vi "imp_test_v10_2.vi"() -> ()   [LabVIEW 2014]
uses:
  <vilib>/LabVIEW Targets/FPGA/cRIO/shared/nicrio_ModuleControls/nicrio_cRIO-9237_DataRatesRing.ctl
  <vilib>/LabVIEW Targets/FPGA/cRIO/shared/nicrio_ModuleControls/nicrio_cRIO-9237_ExcitationVoltageRing.ctl
  <vilib>/rvi/FXPMathLib/FxpSinAndCos/subVIs/nifxpmath_SinAndCos_SimConfig.ctl
  <vilib>/rvi/Emulation/niFpgaGetClockAttributes.vi
  <vilib>/rvi/Emulation/niFpgaSctlEmulationGetInTimedLoop.vi
  <vilib>/rvi/Emulation/niFpgaEmulationReportErrorSimple.vi
  <vilib>/rvi/Emulation/niFpgaProcessEmulError.vi
  <vilib>/rvi/interface/RandomDataEmulation/nirviRandomDataMultiElementFPGAFIFO.vi
  <instcachedir>/0/nirviRandomDataMultiElementFPGAFIFO_AD0CFC12EF974623A9C2E4184BC062B2.lvgen/nirviRandomDataMultiElementFPGAFIFO_AD0CFC12EF974623A9C2E4184BC062B2_010.vi
  <vilib>/rvi/interface/RandomDataEmulation/niFpgaRandomDataHandleErrors.vi
  <vilib>/rvi/Emulation/niFpgaCriticalErrorInLSC.vi
  <vilib>/rvi/FXPMathLib/FxpSinAndCos/simVIs/DllFxpSinAndCosTemp_sub.vi
  <vilib>/rvi/eio/common/nirviEmuTemplateMethod_errors.vi
  <vilib>/rvi/eio/common/nirviEmuTemplatePropertySet_errors.vi
  <vilib>/rvi/DataTransferAndStorage/Container/XNode/niFpgaContainer.xnode
  <vilib>/rvi/interface/RandomDataEmulation/nirviRandomDataFpgaMultiElementTemplate.vi
  <vilib>/rvi/FXPMathLib/FxpSinAndCos/XNode/nifxpmath_SinAndCos.xnode
  <vilib>/eio/EIONode/EIONode.xnode
  <vilib>/rvi/Analysis/measure/butterworth/XNode/niFpgaButterworthFilter.xnode
  <vilib>/eio/EIOPropertyNode/EIOPropertyNode.xnode
  <vilib>/rvi/eio/common/nirviEmuTemplatePropertyGet_errors.vi
  <vilib>/rvi/eio/common/nirviEmuTemplatePropertyGet_noerrors.vi
  <vilib>/rvi/eio/common/nirviEmuTemplatePropertySet_noerrors.vi
panel:
  in  "F_Threshold_p":fxp<+,12,4>
  in  "F_Threshold_y":fxp<+,12,4>
  out "omega_y (Mavg)":fxp<+/-,36,13>
  out "Dy_d (Mavg)":fxp<+/-,36,13>
  out "omega_p (Mavg)":fxp<+/-,36,13>
  out "Dp_d (Mavg)":fxp<+/-,36,13>
  out "omega_p2 (Mavg)":fxp<+/-,36,14>
  out "Dp2_d (Mavg)":fxp<+/-,36,14>
  out "omega_y2 (Mavg)":fxp<+/-,36,14>
  out "Dy2_d (Mavg)":fxp<+/-,36,14>
  in  "mt0_y2":u32
  in  "mt0_p2":u32
  out "Dy_d (Mavg w. f.)":fxp<+/-,36,14>
  out "Dp_d (Mavg w. f.)":fxp<+/-,36,14>
  in  "Dp_d (Mavg) coeff.":i32[](array[numeric])=[946630756, 63555534]
  in  "Dy_d (Mavg) coeff.":i32[](array[numeric])=[946630756, 63555534]
  out "omega_y (Mavg w. f.)":fxp<+/-,36,14>
  in  "omega_y(Mavg) coeff.":i32[](array[numeric])=[946630756, 63555534]
  out "omega_p (Mavg w. f)":fxp<+/-,36,14>
  in  "omega_P(Mavg) coeff.":i32[](array[numeric])=[946630756, 63555534]
  out "PID (kHz)":fxp<+/-,20,10>
  in  "Set 6":bool
  in  "Set 5":bool
  in  "Set 4":bool
  in  "Set 3":bool
  in  "Set 2":bool
  in  "Set 1":bool
  out "Dy1_d (T)":fxp<+/-,36,13>
  out "omega_y1 (T)":fxp<+/-,36,13>
  out "Dp1_d (T)":fxp<+/-,36,13>
  out "omega_p1 (T)":fxp<+/-,36,13>
  out "Dy2_d (T)":fxp<+/-,36,13>
  out "Dp2_d (T)":fxp<+/-,36,13>
  out "omega_y2 (T)":fxp<+/-,36,13>
  out "omega_p2 (T)":fxp<+/-,36,13>
  out "mt_omega_y2":u32
  out "mt_omega_p2":u32
  out "rad_y2":fxp<+/-,33,20>
  out "D_y2":fxp<+/-,32,7>
  out "rad_y1":fxp<+/-,33,20>
  out "D_y1":fxp<+/-,32,7>
  out "Encoder Position_y1":i32
  out "Encoder Position_y2":i32
  out "Encoder Position_p2":i32
  out "D_p2":fxp<+/-,32,7>
  out "rad_p2":fxp<+/-,33,20>
  out "D_p1":fxp<+/-,32,7>
  out "rad_p1":fxp<+/-,33,20>
  out "Encoder Position_p1":i32
  in  "Mag. factor_y":fxp<+/-,20,3>
  in  "Mag. encoder_y":bool
  out "omega_y (rad/s)":fxp<+/-,36,13>
  out "Dy_d (mm/s)":fxp<+/-,36,13>
  in  "Vy. Est.":i16(ring) items=["T", "Mavg", "Mavg w. f."]
  out "omega_y1 (Mavg)":fxp<+/-,36,14>
  out "Dy1_d (Mavg)":fxp<+/-,36,14>
  in  "Dy_d_M_avg_Tc (uSec)":i32
  out "Dp1_d (Mavg)":fxp<+/-,36,14>
  out "omega_p1 (Mavg)":fxp<+/-,36,14>
  in  "Dp_d_M_avg_Tc (uSec)":i32
  out "Dp_d (T)":fxp<+/-,36,13>
  out "omega_p (T)":fxp<+/-,36,13>
  in  "Vp. Est.":i16(ring) items=["T", "Mavg", "Mavg w. f."]
  in  "Mag. factor_p":fxp<+/-,20,3>
  in  "Mag. encoder_p":bool
  in  "Belt_out_p":fxp<+/-,7,7>
  in  "Belt_in_p":fxp<+/-,6,6>
  in  "Belt_out_y":fxp<+/-,7,7>
  in  "Belt_in_y":fxp<+/-,6,6>
  out "Fp_dc":fxp<+/-,32,10>
  out "Fy_dc":fxp<+/-,32,10>
  in  "Zero_y":bool
  in  "Zero_p":bool
  in  "mt0_p1":u32
  in  "Encoder reset":bool
  out "fpt_d":fxp<+/-,36,18>
  out "Dp_error_dd":fxp<+/-,36,16>
  out "Dp_error_d":fxp<+/-,33,8>
  in  "Dp_dd coeff.":i32[](array[numeric])=[946630756, 63555534]
  out "Dp_dd":fxp<+/-,36,25>
  out "dFp_PID":fxp<+/-,36,18>
  in  "dFp_PID coeff.":i32[](array[numeric])=[946630756, 63555534]
  out "fpt_i":fxp<+/-,34,18>
  in  "Bv_p":fxp<+/-,22,8>
  in  "Kv_p":fxp<+/-,22,8>
  out "Dp_error":fxp<+/-,22,7>
  out "Dpr_sin":fxp<+/-,22,7>
  in  "Sin offset_p":fxp<+/-,22,7>
  in  "Sin magnitude_p":fxp<+/-,21,6>
  out "Dpr_sin_dd":fxp<+/-,35,20>
  out "Dpr_sin_d":fxp<+/-,33,15>
  out "Sin omega_p":fxp<+/-,34,9>
  in  "Sin wave freq._p (Hz)":fxp<+/-,32,6>
  in  "Dpr_step":fxp<+/-,22,7>
  out "Dpr_for":fxp<+/-,22,7>
  in  "Command_p":i16(ring) items=["Step", "Sine"]
  in  "Ki_p":fxp<+/-,30,9>
  out "Fp_PID":fxp<+/-,36,16>
  in  "fp_tolorance":fxp<+,22,6>
  out "fp_tilde":fxp<+/-,33,10>
  in  "Kd_p":fxp<+/-,30,9>
  in  "Kp_p":fxp<+/-,32,13>
  out "Fr_p":fxp<+/-,32,10>
  in  "S/F coeff_p":fxp<+/-,25,-10>
  in  "S/F coeff_y":fxp<+/-,25,-10>
  out "va_p":fxp<+/-,36,7>
  out "vb_p":fxp<+/-,37,8>
  out "vq_p_F":fxp<+/-,20,5> format="%.57g"
  out "vd_p_F":fxp<+/-,20,5>
  in  "dFp_add":bool
  in  "Stop motor_p":bool
  out "Force_p":fxp<+/-,32,10>
  in  "Strain selection_p":i16(ring) items=["Raw", "Avg.8", "Avg.8 w. filter"]
  out "Strain_p (Avg8 w. f)":fxp<+/-,36,8>
  in  "Strain_p Avg.8 coeff.":i32[](array[numeric])=[946630756, 63555534]
  out "Strain_p (Avg8)":fxp<+/-,36,4>
  out "Raw Strain_p":fxp<+/-,36,4>
  out "Mod6/AI3":fxp<+/-,36,4>
  in  "Strain gage reset_p":bool
  out "Dp_d (mm/s)":fxp<+/-,36,13>
  out "omega_p (rad/s)":fxp<+/-,36,13>
  out "mt_omega_p1":u32
  out "rad_p(NrTheta)":fxp<+/-,33,20>
  out "D_p(mm)":fxp<+/-,32,7>
  out "Encoder Position_p":i32
  in  "Encoder reset_p":bool
  out "Strain_y (Avg8 w. f)":fxp<+/-,36,8>
  in  "Strain_y Avg8 coeff.":i32[](array[numeric])=[-898916953, 1957103773, 3888751]
  out "Dyr_for":fxp<+/-,22,7>
  in  "Command_y":i16(ring) items=["Step", "Sine"]
  out "Strain_y (Avg8)":fxp<+/-,36,4>
  in  "Strain selection_y":i16(ring) items=["Raw", "Avg.8", "Avg.8 w. filter"]
  out "vb_y":fxp<+/-,38,8>
  out "va_y":fxp<+/-,38,8>
  out "fyt_d":fxp<+/-,36,18>
  out "Fr_y":fxp<+/-,32,10>
  in  "Bv_y":fxp<+/-,22,8>
  out "Dy_error_dd":fxp<+/-,36,16>
  out "Dy_error_d":fxp<+/-,33,8>
  in  "Kv_y":fxp<+/-,22,8>
  out "Dy_error":fxp<+/-,22,7>
  out "Dyr_sin_dd":fxp<+/-,35,20>
  out "Dyr_sin_d":fxp<+/-,33,15>
  out "Sin omega_y":fxp<+/-,34,9>
  out "Dyr_sin":fxp<+/-,22,7>
  in  "Sin offset_y":fxp<+/-,22,7>
  in  "Sin magnitude_y":fxp<+/-,21,6>
  out "Time now(s)":fxp<+,52,14>
  in  "Sin wave freq._y (Hz)":fxp<+/-,32,6>
  in  "Dyr_step":fxp<+/-,22,7>
  in  "Drive mode":i16(ring) items=["Backward", "Forward"]
  out "Dy_dd":fxp<+/-,36,25>
  in  "Dy_dd coeff.":i32[](array[numeric])=[946630756, 63555534]
  out "dFy_PID":fxp<+/-,36,18>
  in  "dFy_PID coeff.":i32[](array[numeric])=[946630756, 63555534]
  out "fyt_i":fxp<+/-,36,16>
  out "Fy_PID":fxp<+/-,36,16>
  in  "fy_tolorance":fxp<+,22,6>
  in  "Ki_y":fxp<+/-,30,9>
  in  "Kd_y":fxp<+/-,30,9>
  out "fy_tilde":fxp<+/-,32,10>
  in  "Kp_y":fxp<+/-,32,13>
  out "vq_y_F":fxp<+/-,20,5> format="%.57g"
  out "vd_y_F":fxp<+/-,20,5>
  in  "dFy_add":bool
  in  "Stop motor_y":bool
  out "Dy_d (T)":fxp<+/-,36,13>
  out "omega_y (T)":fxp<+/-,36,13>
  in  "mt0_y1":u32
  out "mt_omega_y1":u32
  out "rad_y(NrTheta)":fxp<+/-,33,20>
  out "D_y(mm)":fxp<+/-,32,7>
  out "Encoder Position_y":i32
  in  "Encoder reset_y":bool
  in  "Ini coe.":bool
  out "Loop rate (kHz)":fxp<+/-,36,7>
  out "Force_y":fxp<+/-,32,10>
  out "Raw Strain_y":fxp<+/-,36,4>
  in  "Strain gage reset_y":bool
  in  "Stop (Strain)":bool
  out "Mod6/AI2":fxp<+/-,36,4>
  in  "Excitation Voltage":T1 items=["2.5 Volts", "3.3 Volts", "5.0 Volts", "10.0 Volts", "External Excitation"]
  in  "Data Rate":T2=1 items=["50.000 kS/s (NI 9237)"=1, "25.000 kS/s (NI 9237)"=2, "16.667 kS/s (NI 9237)"=3, "12.500 kS/s (NI 9237)"=4, "10.000 kS/s (NI 9237)"=5, "8.333 kS/s (NI 9237)"=6, "7.143 kS/s (NI 9237)"=7, "6.250 kS/s (NI 9237)"=8, "5.556 kS/s (NI 9237)"=9, "5.000 kS/s (NI 9237)"=10, "4.545 kS/s (NI 9237)"=11, "4.167 kS/s (NI 9237)"=12, "3.846 kS/s (NI 9237)"=13, "3.571 kS/s (NI 9237)"=14, "3.333 kS/s (NI 9237)"=15, "3.125 kS/s (NI 9237)"=16, "2.941 kS/s (NI 9237)"=17, "2.778 kS/s (NI 9237)"=18, "2.632 kS/s (NI 9237)"=19, "2.500 kS/s (NI 9237)"=20, "2.381 kS/s (NI 9237)"=21, "2.273 kS/s (NI 9237)"=22, "2.174 kS/s (NI 9237)"=23, "2.083 kS/s (NI 9237)"=24, "2.000 kS/s (NI 9237)"=25, "1.923 kS/s (NI 9237)"=26, "1.852 kS/s (NI 9237)"=27, "1.786 kS/s (NI 9237)"=28, "1.724 kS/s (NI 9237)"=29, "1.667 kS/s (NI 9237)"=30, "1.613 kS/s (NI 9237)"=31]
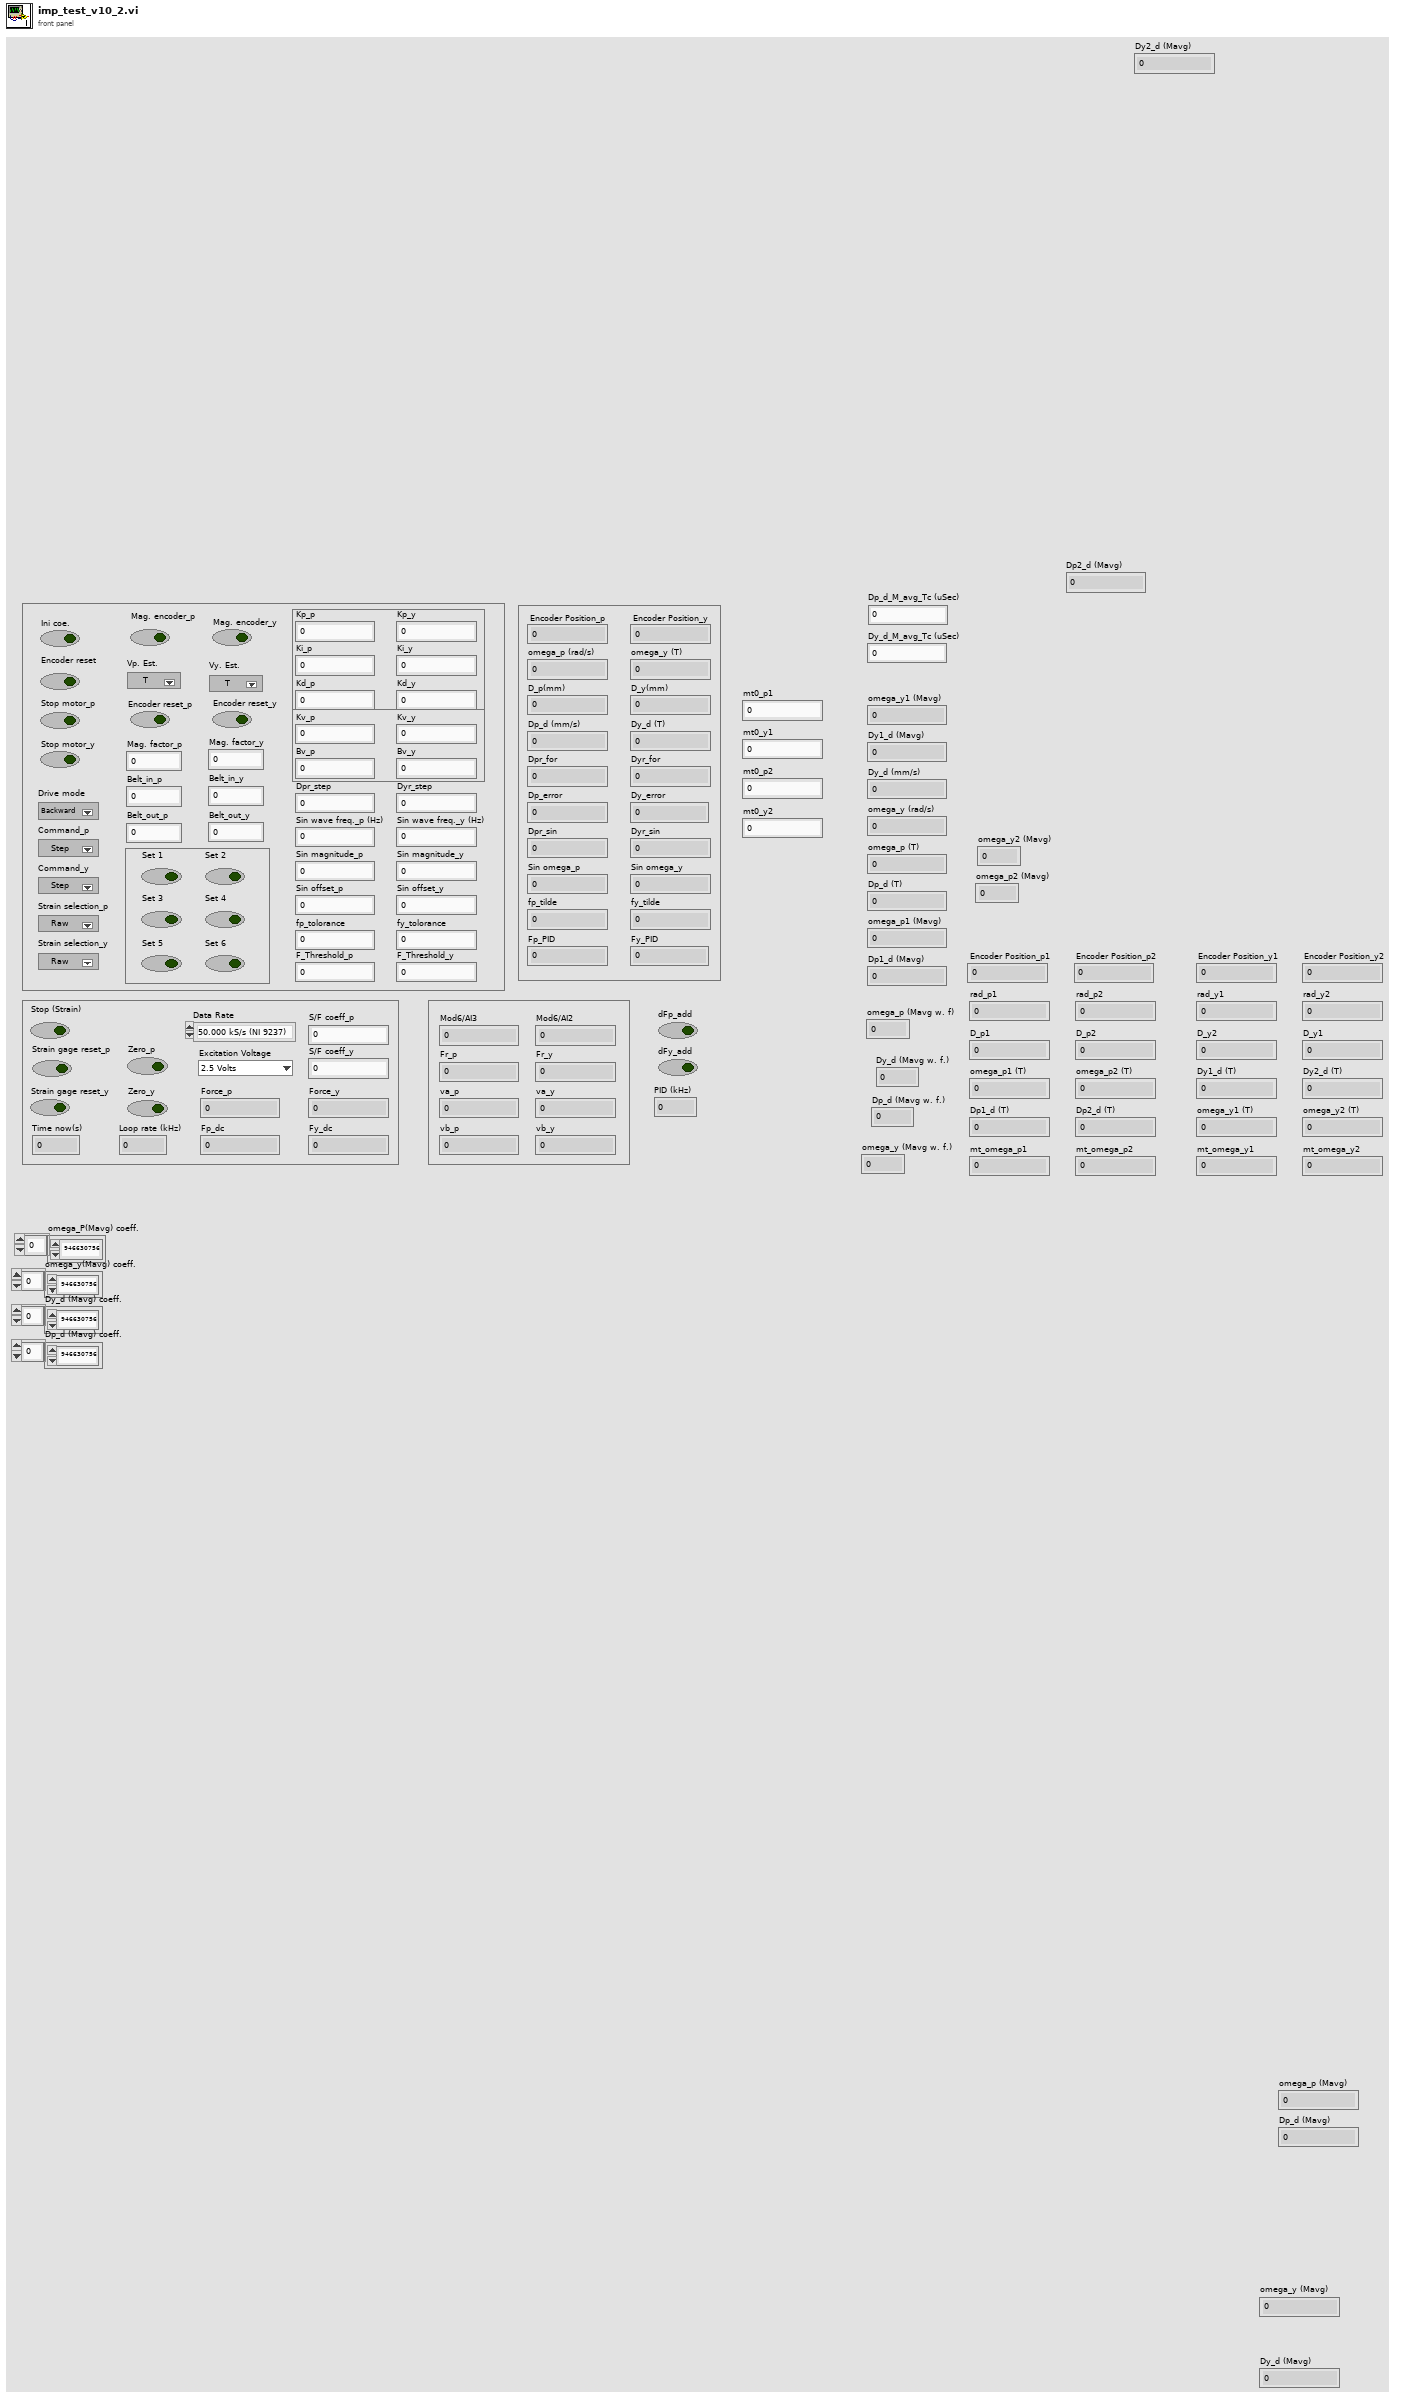
[diagram p1: front panel]
types:
  T1 = typedef "nicrio_cRIO-9237_ExcitationVoltageRing.ctl" = u8
  T2 = typedef "nicrio_cRIO-9237_DataRatesRing.ctl" = u8
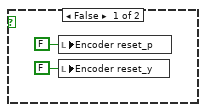
[diagram p12: hidden frame]
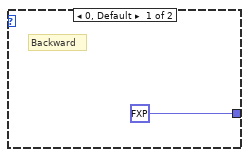
[diagram p13: hidden frame]
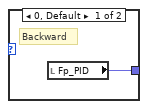
[diagram p14: hidden frame]
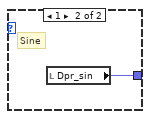
[diagram p15: hidden frame]
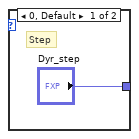
[diagram p16: hidden frame]
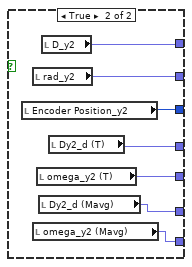
[diagram p17: hidden frame]
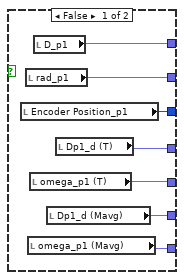
[diagram p18: hidden frame]
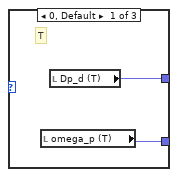
[diagram p19: hidden frame]
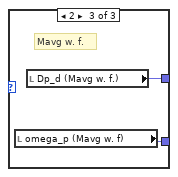
[diagram p20: hidden frame]
diagram:
  w2 = 25
  w5 = i16 25
  w13 = 25
  w16 = 25
  w21 = TRUE ("Half-Bridge Enable")
  # "rad_x2那邊:數據叫出來/8才會和馬達編碼器的rad一樣??"
  # "Encoder 4096ppr\nomega = 61359.2315154/mt\nomega0 = 2*pi/4096 (rad/s)"
  # "Encoder 800ppr\nomega = 314159.265359/mt\nomega0 = 2*pi/800 (rad/s)"
  # "v9\nKp改32/13\nKd改30/9\nKo改30/9"
  # "Resolutuin of Mag. Encoder = 4096*(F_mag)"
  # "use Mavg method to estimate omega or velocity from magnetic encoder"
  # "為什麼要寫兩個迴圈?\nv9後已修正"
  # "Dr_dd ?"
  # "Dr_d ?"
  n1 = xnode "FPGA I/O Property Node"("error in"=errorcluster {"status"=FALSE, "code"=0, "source"=""}, "Data Rate"="Data Rate", "Excitation Voltage"="Excitation Voltage") -> ("error out"=w26:errorcluster)  [unwired: 1 in, 1 out]
  n2 = xnode "FPGA I/O Property Node"("error in"=w26, "Half-Bridge Enable"=w21) -> ("error out"=w19:errorcluster)  [unwired: 1 in, 1 out]
  n3 = xnode "FPGA I/O Property Node"("Half-Bridge Enable"=w21) -> ("error out"=w18:errorcluster)  [unwired: 2 in, 1 out]
  n4 = Merge Errors(w19, w18) -> (w20:errorcluster)
  n5 = xnode "FPGA I/O Node"("error in"=w20, "Mod6/Start"=TRUE) -> ("error out"=w24:errorcluster)  [unwired: 1 in, 1 out]
  n6 = while "AO_p" {
    stop <- FALSE stop-if-true
    n7 = flat-sequence {
      frame #0 {
        n8 = local read "rad_p(NrTheta)"() -> (w41:fxp<+/-,33,20>)
        n9 = local read "vq_p_F"() -> (w42:fxp<+/-,20,5>)
        n10 = local read "vd_p_F"() -> (w44:fxp<+/-,20,5>)
        n11 = Select(t=fxp<+/-,20,5> 0.0, s="Stop motor_p", f=w44) -> (s? t:f=w33:fxp<+/-,20,5>)
        n12 = Select(t=fxp<+,1,1> 0.0, s="Stop motor_p", f=w42) -> (s? t:f=w32:fxp<+/-,20,5>)
        n13 = xnode "High Throughput Sine & Cosine"("x (pi)"=w41) -> ("sin(x)"=w35:fxp<+/-,16,2>, "cos(x)"=w34:fxp<+/-,16,2>)
        n14 = Negate(x=w32) -> (-x=w40:fxp<+/-,21,6>)
        n15 = Multiply(x=w33, y=w35) -> (x*y=w39:fxp<+/-,36,7>)
        n16 = Multiply(x=w33, y=w34) -> (x*y=w37:fxp<+/-,36,7>)
        n17 = Multiply(x=w34, y=w32) -> (x*y=w38:fxp<+/-,36,7>)
        n18 = Multiply(x=w35, y=w40) -> (x*y=w36:fxp<+/-,35,6>)
        n19 = Add(x=w39, y=w38) -> (x+y=→"vb_p":fxp<+/-,37,8>)
        n20 = Add(x=w37, y=w36) -> (x+y=→"va_p":fxp<+/-,36,7>)
      }
      frame #1 {
        n21 = local read "Encoder reset_p"() -> (w77:bool)
        n22 = local read "vb_p"() -> (w78:fxp<+/-,37,8>)
        n23 = local read "va_p"() -> (w79:fxp<+/-,36,7>)
        n24 = Select(t=fxp<+,2,2> 3.0, s=w77, f=w79) -> (s? t:f=w85:fxp<+/-,36,7>)
        n25 = Select(t=fxp<+,1,1> 0.0, s=w77, f=w78) -> (s? t:f=w84:fxp<+/-,37,8>)
        n26 = Multiply(x=w85, y=fxp<+/-,1,0> -0.5) -> (x*y=w80:fxp<+/-,36,6>)
        n27 = Multiply(x=w84, y=fxp<+/-,1,0> -0.5) -> (x*y=w81:fxp<+/-,36,6>)
        n28 = xnode "FPGA I/O Node"("Mod8/AO0"=w80, "Mod8/AO1"=w81) -> ()  [unwired: 2 in, 2 out]
      }
    }
  }
  n29 = while "AO_y" {
    stop <- FALSE stop-if-true
    n30 = flat-sequence {
      frame #0 {
        n31 = local read "rad_y(NrTheta)"() -> (w105:fxp<+/-,33,20>)
        n32 = local read "vd_y_F"() -> (w103:fxp<+/-,20,5>)
        n33 = local read "vq_y_F"() -> (w102:fxp<+/-,20,5>)
        n34 = Select(t=fxp<+/-,20,5> 0.0, s="Stop motor_y", f=w103) -> (s? t:f=w97:fxp<+/-,20,5>)
        n35 = Select(t=fxp<+/-,20,5> 0.0, s="Stop motor_y", f=w102) -> (s? t:f=w96:fxp<+/-,20,5>)
        n36 = xnode "High Throughput Sine & Cosine"("x (pi)"=w105) -> ("sin(x)"=w99:fxp<+/-,17,2>, "cos(x)"=w98:fxp<+/-,17,2>)
        n37 = Negate(x=w96) -> (-x=w95:fxp<+/-,21,6>)
        n38 = Multiply(x=w97, y=w99) -> (x*y=w94:fxp<+/-,37,7>)
        n39 = Multiply(x=w97, y=w98) -> (x*y=w92:fxp<+/-,37,7>)
        n40 = Multiply(x=w98, y=w96) -> (x*y=w93:fxp<+/-,37,7>)
        n41 = Multiply(x=w99, y=w95) -> (x*y=w91:fxp<+/-,36,6>)
        n42 = Add(x=w94, y=w93) -> (x+y=→"vb_y":fxp<+/-,38,8>)
        n43 = Add(x=w92, y=w91) -> (x+y=→"va_y":fxp<+/-,37,7>)
      }
      frame #1 {
        n44 = local read "Encoder reset_y"() -> (w138:bool)
        n45 = local read "va_y"() -> (w137:fxp<+/-,38,8>)
        n46 = local read "vb_y"() -> (w136:fxp<+/-,38,8>)
        n47 = Select(t=fxp<+,2,2> 3.0, s=w138, f=w137) -> (s? t:f=w142:fxp<+/-,38,8>)
        n48 = Select(t=fxp<+,1,1> 0.0, s=w138, f=w136) -> (s? t:f=w141:fxp<+/-,38,8>)
        n49 = Multiply(x=w142, y=fxp<+/-,1,0> -0.5) -> (x*y=w145:fxp<+/-,39,8>)
        n50 = Multiply(x=w141, y=fxp<+/-,1,0> -0.5) -> (x*y=w146:fxp<+/-,37,6>)
        n51 = xnode "FPGA I/O Node"("Mod8/AO2"=w145, "Mod8/AO3"=w146) -> ()  [unwired: 2 in, 2 out]
      }
    }
  }
  n52 = while "Selection" {
    stop <- FALSE stop-if-true
    # "T = Mag. encoder\nF = Motor encoder"
    n53 = case shown="2" "Strain selection_y" {
      tunnel: [w229 w230 w231] -> w182
      frame 0, Default {
        n54 = local read "Raw Strain_y"() -> (w229:fxp<+/-,36,4>)
      }
      frame 1 {
        n55 = local read "Strain_y (Avg8)"() -> (w230:fxp<+/-,36,4>)
      }
      frame 2 {
        n56 = local read "Strain_y (Avg8 w. f)"() -> (w231:fxp<+/-,36,8>)
      }
    }
    n57 = case shown="1" "Vp. Est." {
      tunnel: [w213 w214 w217] -> w165
      tunnel: [w212 w215 w216] -> w166
      frame 0, Default {
        # "T"
        n58 = local read "omega_p (T)"() -> (w213:fxp<+/-,36,13>)
        n59 = local read "Dp_d (T)"() -> (w212:fxp<+/-,36,13>)
      }
      frame 1 {
        # "Mavg"
        n60 = local read "omega_p (Mavg)"() -> (w214:fxp<+/-,36,13>)
        n61 = local read "Dp_d (Mavg)"() -> (w215:fxp<+/-,36,13>)
      }
      frame 2 {
        # "Mavg w. f."
        n62 = local read "omega_p (Mavg w. f)"() -> (w217:fxp<+/-,36,14>)
        n63 = local read "Dp_d (Mavg w. f.)"() -> (w216:fxp<+/-,36,14>)
      }
    }
    "Dp_d (mm/s)" <- w166
    "omega_p (rad/s)" <- w165
    n64 = Divide(x=w182, y="S/F coeff_y") -> (x/y=w175:fxp<+/-,32,10>)
    n65 = case shown="True" "Zero_y" {
      tunnel: w175 -> [_ w225]
      frame False {
      }
      frame True {
        "Fy_dc" <- w225
      }
    }
    n66 = local read "Fy_dc"() -> (w176:fxp<+/-,32,10>)
    n67 = Subtract(x=w175, y=w176) -> (x-y=→"Force_y":fxp<+/-,33,11>)
    n68 = case shown="2" "Strain selection_p" {
      tunnel: [w226 w227 w228] -> w180
      frame 0, Default {
        n69 = local read "Raw Strain_p"() -> (w226:fxp<+/-,36,4>)
      }
      frame 1 {
        n70 = local read "Strain_p (Avg8)"() -> (w227:fxp<+/-,36,4>)
      }
      frame 2 {
        n71 = local read "Strain_p (Avg8 w. f)"() -> (w228:fxp<+/-,36,8>)
      }
    }
    n72 = case shown="1" "Vy. Est." {
      tunnel: [w219 w221 w223] -> w168
      tunnel: [w218 w220 w222] -> w169
      frame 0, Default {
        # "T"
        n73 = local read "omega_y (T)"() -> (w218:fxp<+/-,36,13>)
        n74 = local read "Dy_d (T)"() -> (w219:fxp<+/-,36,13>)
      }
      frame 1 {
        # "Mavg"
        n75 = local read "omega_y (Mavg)"() -> (w220:fxp<+/-,36,13>)
        n76 = local read "Dy_d (Mavg)"() -> (w221:fxp<+/-,36,13>)
      }
      frame 2 {
        # "Mavg w. f."
        n77 = local read "omega_y (Mavg w. f.)"() -> (w222:fxp<+/-,36,14>)
        n78 = local read "Dy_d (Mavg w. f.)"() -> (w223:fxp<+/-,36,14>)
      }
    }
    "Dy_d (mm/s)" <- w168
    "omega_y (rad/s)" <- w169
    n79 = Divide(x=w180, y="S/F coeff_p") -> (x/y=w172:fxp<+/-,32,10>)
    n80 = case shown="True" "Zero_p" {
      tunnel: w172 -> [_ w224]
      frame False {
      }
      frame True {
        "Fp_dc" <- w224
      }
    }
    n81 = local read "Fp_dc"() -> (w170:fxp<+/-,32,10>)
    n82 = Subtract(x=w172, y=w170) -> (x-y=→"Force_p":fxp<+/-,33,11>)
    n83 = case shown="False" "Mag. encoder_y" {
      tunnel: [w190 w196] -> w156
      tunnel: [w189 w197] -> w157
      tunnel: [w188 w195] -> w159
      tunnel: [w186 w194] -> w153
      tunnel: [w187 w193] -> w152
      tunnel: [w185 w192] -> w148
      tunnel: [w184 w191] -> w147
      frame False {
        n84 = local read "Encoder Position_y1"() -> (w188:i32)
        n85 = local read "omega_y1 (Mavg)"() -> (w184:fxp<+/-,36,14>)
        n86 = local read "Dy1_d (Mavg)"() -> (w185:fxp<+/-,36,14>)
        n87 = local read "rad_y1"() -> (w190:fxp<+/-,33,20>)
        n88 = local read "omega_y1 (T)"() -> (w186:fxp<+/-,36,13>)
        n89 = local read "D_y1"() -> (w189:fxp<+/-,32,7>)
        n90 = local read "Dy1_d (T)"() -> (w187:fxp<+/-,36,13>)
      }
      frame True {
        n91 = local read "Encoder Position_y2"() -> (w195:i32)
        n92 = local read "rad_y2"() -> (w196:fxp<+/-,33,20>)
        n93 = local read "omega_y2 (Mavg)"() -> (w191:fxp<+/-,36,14>)
        n94 = local read "omega_y2 (T)"() -> (w194:fxp<+/-,36,13>)
        n95 = local read "Dy2_d (Mavg)"() -> (w192:fxp<+/-,36,14>)
        n96 = local read "D_y2"() -> (w197:fxp<+/-,32,7>)
        n97 = local read "Dy2_d (T)"() -> (w193:fxp<+/-,36,13>)
      }
    }
    "D_y(mm)" <- w157
    "rad_y(NrTheta)" <- w156
    "Encoder Position_y" <- w159
    "Dy_d (T)" <- w152
    "omega_y (T)" <- w153
    "Dy_d (Mavg)" <- w148
    "omega_y (Mavg)" <- w147
    n98 = case shown="True" "Mag. encoder_p" {
      tunnel: [w204 w211] -> w161
      tunnel: [w203 w210] -> w162
      tunnel: [w202 w209] -> w163
      tunnel: [w200 w208] -> w155
      tunnel: [w201 w207] -> w154
      tunnel: [w199 w205] -> w151
      tunnel: [w198 w206] -> w150
      frame False {
        n99 = local read "Encoder Position_p1"() -> (w202:i32)
        n100 = local read "rad_p1"() -> (w203:fxp<+/-,33,20>)
        n101 = local read "omega_p1 (Mavg)"() -> (w198:fxp<+/-,36,14>)
        n102 = local read "omega_p1 (T)"() -> (w200:fxp<+/-,36,13>)
        n103 = local read "D_p1"() -> (w204:fxp<+/-,32,7>)
        n104 = local read "Dp1_d (Mavg)"() -> (w199:fxp<+/-,36,14>)
        n105 = local read "Dp1_d (T)"() -> (w201:fxp<+/-,36,13>)
      }
      frame True {
        n106 = local read "Encoder Position_p2"() -> (w209:i32)
        n107 = local read "omega_p2 (Mavg)"() -> (w206:fxp<+/-,36,14>)
        n108 = local read "rad_p2"() -> (w210:fxp<+/-,33,20>)
        n109 = local read "D_p2"() -> (w211:fxp<+/-,32,7>)
        n110 = local read "Dp2_d (Mavg)"() -> (w205:fxp<+/-,36,14>)
        n111 = local read "omega_p2 (T)"() -> (w208:fxp<+/-,36,13>)
        n112 = local read "Dp2_d (T)"() -> (w207:fxp<+/-,36,13>)
      }
    }
    "D_p(mm)" <- w161
    "rad_p(NrTheta)" <- w162
    "Encoder Position_p" <- w163
    "Dp_d (T)" <- w154
    "omega_p (T)" <- w155
    "Dp_d (Mavg)" <- w151
    "omega_p (Mavg)" <- w150
  }
  n113 = while "Quadrature drive_y" {
    stop <- FALSE stop-if-true
    n114 = local read "Drive mode"() -> (w233:i16)
    n115 = case shown="1" w233 {
      tunnel: [w243 w244] -> w232
      frame 0, Default {
        # "Backward"
        n116 = local read "Fy_PID"() -> (w243:fxp<+/-,36,16>)
      }
      frame 1 {
        # "Forward"
        n117 = local read "Fr_y"() -> (w244:fxp<+/-,32,10>)
      }
    }
    n118 = local read "dFy_PID"() -> (w236:fxp<+/-,36,18>)
    n119 = local read "omega_y (rad/s)"() -> (w242:fxp<+/-,36,13>)
    n120 = Select(t=w236, s="dFy_add", f=fxp<+,1,1> 0.0) -> (s? t:f=w239:fxp<+/-,36,18>)
    n121 = call "Oriental_step_motor_PKP225.vi"("F_Threshold"="F_Threshold_y", "dFmr"=w239, "omega"=w242, "Fmr"=w232) -> ("vq_F"=→"vq_y_F":fxp<+/-,36,9>, "vd_F"=→"vd_y_F":fxp<+/-,36,9>)  [unwired: 6 in]
  }
  n122 = while "Encoder_p" {
    shift-right: [w282] -> _
    shift-left: _ -> [w281]
    shift-right: [w283] -> _
    shift-left: _ -> [w280]
    shift-right: [w277] -> _
    shift-left: _ -> [w279]
    shift-right: [w268] -> _
    shift-left: _ -> [w267]
    shift-right: [w269] -> _
    shift-left: _ -> [w270]
    shift-right: [w264] -> _
    shift-left: _ -> [w265]
    stop <- FALSE stop-if-true
    w260 = fxp<+/-,20,-5> 0.00048828125  # L/4096
    w258 = fxp<+/-,16,1> 0.0244140625  # 2*50/4096
    w276 = fxp<+/-,20,-5> 0.002499997615814209  # L/800
    w250 = fxp<+/-,16,1> 0.125  # 2*50/800
    n123 = xnode "FPGA I/O Node"() -> ("Mod7/DIO0"=w285:bool, "Mod7/DIO1"=w284:bool)  [unwired: 2 in, 2 out]
    n124 = xnode "FPGA I/O Node"() -> ("Mod7/DIO4"=w272:bool, "Mod7/DIO5"=w271:bool)  [unwired: 2 in, 2 out]
    n125 = local read "Encoder reset_p"() -> (w266:bool)
    n126 = call "encoder_sub.vi"("A_pre"=w281, "B_pre"=w280, "Encoder Position_pre"=w279, "A input"=w285, "Encoder Position Reset"="Encoder reset_p", "B input"=w284) -> ("A"=w282:bool, "B"=w283:bool, "Encoder Position (Counts)"=w277:i32)  [unwired: 19 in]
    "Encoder Position_p1" <- w277
    n127 = call "encoder_sub.vi"("A_pre"=w267, "B_pre"=w270, "Encoder Position_pre"=w265, "A input"=w272, "Encoder Position Reset"=w266, "B input"=w271) -> ("A"=w268:bool, "B"=w269:bool, "Encoder Position (Counts)"=w264:i32)  [unwired: 19 in]
    "Encoder Position_p2" <- w264
    n128 = local read "Belt_in_p"() -> (w275:fxp<+/-,6,6>)
    n129 = local read "Belt_in_p"() -> (w261:fxp<+/-,6,6>)
    n130 = local read "Belt_out_p"() -> (w273:fxp<+/-,7,7>)
    n131 = To Fixed-Point(number=w264) -> (fixed-point=w246:fxp<+/-,32,32>)  [unwired: 1 in]
    n132 = To Fixed-Point(number=w277) -> (fixed-point=w251:fxp<+/-,32,32>)  [unwired: 1 in]
    n133 = local read "Belt_out_p"() -> (w263:fxp<+/-,7,7>)
    n134 = local read "Mag. factor_p"() -> (w257:fxp<+/-,20,3>)
    n135 = Divide(x=w260, y="Mag. factor_p") -> (x/y=w259:fxp<+/-,41,13>)
    n136 = Multiply(x=w276, y=w275) -> (x*y=w274:fxp<+/-,26,1>)
    n137 = Multiply(x=w259, y=w261) -> (x*y=w262:fxp<+/-,46,18>)
    n138 = Divide(x=w274, y=w273) -> (x/y=w253:fxp<+/-,33,1>)
    n139 = Divide(x=w262, y=w263) -> (x/y=w248:fxp<+/-,53,18>)
    n140 = Divide(x=w258, y=w257) -> (x/y=w245:fxp<+/-,37,5>)
    n141 = Multiply(x=w251, y=w250) -> (x*y=→"rad_p1":fxp<+/-,33,20>)
    n142 = Multiply(x=w248, y=w246) -> (x*y=→"D_p2":fxp<+/-,37,7>)
    n143 = Multiply(x=w246, y=w245) -> (x*y=→"rad_p2":fxp<+/-,46,16>)
    n144 = Multiply(x=w253, y=w251) -> (x*y=→"D_p1":fxp<+/-,32,7>)
  }
  n145 = while "Integral and derivative" {
    shift-right: [w341] -> _
    shift-left: _ -> [w340]
    shift-right: [w333] -> _
    shift-left: _ -> [w332]
    shift-right: [w343] -> _
    shift-left: _ -> [w344]
    shift-right: [w323] -> _
    shift-left: _ -> [w322]
    shift-right: [w309] -> _
    shift-left: _ -> [w312]
    shift-right: [w302] -> _
    shift-left: _ -> [w301]
    shift-right: [w296] -> _
    shift-left: _ -> [w295]
    shift-right: [w291] -> _
    shift-left: _ -> [w292]
    stop <- FALSE stop-if-true
    # "Pitch"
    # "Yaw"
    n146 = local read "Dp_d (mm/s)"() -> (w291:fxp<+/-,36,13>)
    n147 = local read "Dy_d (mm/s)"() -> (w323:fxp<+/-,36,13>)
    n148 = local read "Fp_PID"() -> (w296:fxp<+/-,36,16>)
    n149 = local read "fp_tilde"() -> (w313:fxp<+/-,33,10>)
    n150 = local read "fp_tolorance"() -> (w316:fxp<+,22,6>)
    n151 = local read "fy_tolorance"() -> (w319:fxp<+,22,6>)
    n152 = local read "fy_tilde"() -> (w345:fxp<+/-,32,10>)
    n153 = local read "Fy_PID"() -> (w343:fxp<+/-,36,16>)
    n154 = Subtract(x=w296, y=w295) -> (x-y=w300:fxp<+/-,37,17>)
    n155 = Subtract(x=w291, y=w292) -> (x-y=w293:fxp<+/-,37,14>)
    n156 = Absolute Value(x=w313) -> (abs(x)=w317:fxp<+,33,10>)
    n157 = Absolute Value(x=w345) -> (abs(x)=w347:fxp<+,32,10>)
    n158 = Subtract(x=w343, y=w344) -> (x-y=w331:fxp<+/-,37,17>)
    n159 = Subtract(x=w323, y=w322) -> (x-y=w325:fxp<+/-,36,11>)
    n160 = Greater?(x=w347, y=w319) -> (0:w348:bool)
    n161 = Greater?(x=w317, y=w316) -> (0:w315:bool)
    n162 = Multiply(x=fxp<+,7,10> 1000.0, y=w300) -> (x*y=w298:fxp<+/-,32,18>)
    n163 = Multiply(x=fxp<+,7,10> 1000.0, y=w293) -> (x*y=w289:fxp<+/-,36,21>)
    n164 = local read "Stop motor_y"() -> (w334:bool)
    n165 = local read "Stop motor_p"() -> (w304:bool)
    n166 = Select(t=w345, s=w348, f=fxp<+/-,33,11> 0.0) -> (s? t:f=w341:fxp<+/-,33,11>)
    n167 = Select(t=w313, s=w315, f=fxp<+,1,1> 0.0) -> (s? t:f=w309:fxp<+/-,33,10>)
    n168 = Multiply(x=fxp<+,7,10> 1000.0, y=w325) -> (x*y=w324:fxp<+/-,36,21>)
    n169 = xnode "Butterworth Filter"("input data"=w298, "scaled coefficients"="dFp_PID coeff.") -> ("output data"=→"dFp_PID":fxp<+/-,36,22>)  [unwired: 1 in]
    n170 = xnode "Butterworth Filter"("input data"=w289, "scaled coefficients"="Dp_dd coeff.") -> ("output data"=→"Dp_dd":fxp<+/-,36,25>)  [unwired: 1 in]
    n171 = Multiply(x=fxp<+,7,10> 1000.0, y=w331) -> (x*y=w328:fxp<+/-,32,18>)
    n172 = Add(x=w340, y=w341) -> (x+y=w346:fxp<+/-,34,12>)
    n173 = Multiply(x=w312, y=w309) -> (x*y=w311:fxp<+/-,34,12>)
    n174 = xnode "Butterworth Filter"("input data"=w324, "scaled coefficients"="Dy_dd coeff.") -> ("output data"=→"Dy_dd":fxp<+/-,36,25>)  [unwired: 1 in]
    n175 = Multiply(x=fxp<+/-,30,12> 0.000499725341796875, y=w346) -> (x*y=w339:fxp<+/-,34,10>)
    n176 = Multiply(x=fxp<+/-,30,12> 0.000499725341796875, y=w311) -> (x*y=w308:fxp<+/-,34,10>)
    n177 = xnode "Butterworth Filter"("input data"=w328, "scaled coefficients"="dFy_PID coeff.") -> ("output data"=→"dFy_PID":fxp<+/-,36,22>)  [unwired: 1 in]
    n178 = Select(t=fxp<+,1,1> 0.0, s=w334, f=fxp<+,1,1> 1.0) -> (s? t:f=w337:fxp<+,1,1>)
    n179 = Select(t=fxp<+,1,1> 0.0, s=w304, f=fxp<+,1,1> 1.0) -> (s? t:f=w306:fxp<+,1,1>)
    n180 = Add(x=w339, y=w332) -> (x+y=w338:fxp<+/-,36,16>)
    n181 = Add(x=w308, y=w301) -> (x+y=w307:fxp<+/-,36,16>)
    n182 = Multiply(x=w338, y=w337) -> (x*y=w333:fxp<+/-,34,18>)
    "fyt_i" <- w333
    n183 = Multiply(x=w307, y=w306) -> (x*y=w302:fxp<+/-,34,18>)
    "fpt_i" <- w302
    n184 = call "Wait"("Count(uSec)"=u32 1000) -> ()  [unwired: 1 out]
  }
  n185 = while {
    stop <- FALSE stop-if-true
    n186 = case shown="True" "Set 3" {
      frame False {
      }
      frame True {
        n187 = local write "fp_tolorance"(fxp<+,22,6> 3.0 ("fp_tolorance")) -> ()
        n188 = local write "Kp_p"(fxp<+/-,36,9> 100.0 ("Kp_p")) -> ()
      }
    }
    n189 = case shown="True" "Set 2" {
      frame False {
      }
      frame True {
        n190 = local write "fp_tolorance"(fxp<+,22,6> 1.5 ("fp_tolorance")) -> ()
        n191 = local write "Kp_p"(fxp<+/-,36,9> 50.0 ("Kp_p")) -> ()
      }
    }
    n192 = case shown="True" "Set 1" {
      frame False {
      }
      frame True {
        n193 = local write "fp_tolorance"(fxp<+,22,6> 3.0 ("fp_tolorance")) -> ()
        n194 = local write "Kp_p"(fxp<+/-,36,9> 50.0 ("Kp_p")) -> ()
      }
    }
    n195 = case shown="True" "Set 5" {
      frame False {
      }
      frame True {
        n196 = local write "fp_tolorance"(fxp<+,22,6> 3.0 ("fp_tolorance")) -> ()
        n197 = local write "Kp_p"(fxp<+/-,36,9> 150.0 ("Kp_p")) -> ()
      }
    }
    n198 = case shown="True" "Set 6" {
      frame False {
      }
      frame True {
        n199 = local write "fp_tolorance"(fxp<+,22,6> 1.5 ("fp_tolorance")) -> ()
        n200 = local write "Kp_p"(fxp<+/-,36,9> 150.0 ("Kp_p")) -> ()
      }
    }
    n201 = case shown="True" "Set 4" {
      frame False {
      }
      frame True {
        n202 = local write "fp_tolorance"(fxp<+,22,6> 1.5 ("fp_tolorance")) -> ()
        n203 = local write "Kp_p"(fxp<+/-,36,9> 100.0 ("Kp_p")) -> ()
      }
    }
  }
  n204 = while "Omega_p(T method)" {
    shift-right: [w432] -> _
    shift-left: _ -> [w430]
    shift-right: [w413] -> _
    shift-left: _ -> [w431]
    shift-right: [w428] -> _
    shift-left: _ -> [w429]
    shift-right: [w406] -> _
    shift-left: _ -> [w405]
    shift-right: [w401] -> _
    shift-left: _ -> [w403]
    shift-right: [w409] -> _
    shift-left: _ -> [w408]
    stop <- FALSE stop-if-true
    w420 = fxp<+/-,32,0> 0.3183098859153688  # L/2/pi
    w425 = fxp<+/-,32,0> 0.3183098859153688  # L/2/pi
    n205 = local read "Encoder Position_p1"() -> (w432:i32)
    n206 = local read "Encoder Position_p2"() -> (w406:i32)
    n207 = call "Tick Count4"() -> ("Tick Count(Ticks)"=w407:u32)
    n208 = call "omega_sub_Encoder_800ppr.vi"("mt0"="mt0_p1", "omega_pre"=w431, "ticks_m_pre"=w429, "ticks"=w407, "count_pre"=w430, "count"=w432) -> ("ticks_m"=w428:u32, "mt"=→"mt_omega_p1":u32, "omega"=w413:fxp<+/-,36,13>)  [unwired: 3 in]
    "omega_p1 (T)" <- w413
    n209 = call "omega_sub_Encoder_4096ppr.vi"("mt0"="mt0_p2", "omega_pre"=w403, "ticks_m_pre"=w408, "ticks"=w407, "count_pre"=w405, "count"=w406) -> ("ticks_m"=w409:u32, "mt"=→"mt_omega_p2":u32, "omega"=w401:fxp<+/-,36,13>)  [unwired: 3 in]
    n210 = local read "Mag. factor_p"() -> (w421:fxp<+/-,20,3>)
    n211 = local read "Belt_in_p"() -> (w418:fxp<+/-,6,6>)
    n212 = local read "Belt_out_p"() -> (w417:fxp<+/-,7,7>)
    n213 = Multiply(x=w425, y="Belt_in_p") -> (x*y=w423:fxp<+/-,38,6>)
    n214 = Multiply(x=w420, y=w418) -> (x*y=w419:fxp<+/-,38,6>)
    n215 = Divide(x=w423, y="Belt_out_p") -> (x/y=w414:fxp<+/-,20,1>)
    n216 = Divide(x=w401, y=w421) -> (x/y=w402:fxp<+/-,57,31>)
    "omega_p2 (T)" <- w402
    n217 = Divide(x=w419, y=w417) -> (x/y=w412:fxp<+/-,45,6>)
    n218 = Multiply(x=w412, y=w402) -> (x*y=→"Dp2_d (T)":fxp<+/-,36,13>)
    n219 = Multiply(x=w414, y=w413) -> (x*y=→"Dp1_d (T)":fxp<+/-,36,13>)
  }
  n220 = while "PD position controller_y" {
    stop <- FALSE stop-if-true
    n221 = case shown="1" "Drive mode" {
      tunnel: [fxp<+/-,62,19> 0.0 w438] -> w434
      frame 0, Default {
        # "Backward"
      }
      frame 1 {
        # "Forward"
        n222 = local read "Dy_error_d"() -> (w440:fxp<+/-,33,8>)
        n223 = local read "D_y(mm)"() -> (w445:fxp<+/-,32,7>)
        n224 = local read "Dyr_for"() -> (w437:fxp<+/-,22,7>)
        n225 = Subtract(x=w437, y=w445) -> (x-y=w444:fxp<+/-,33,8>)
        "Dy_error" <- w444
        n226 = Multiply(x=w444, y="Kv_y") -> (x*y=w442:fxp<+/-,54,15>)
        n227 = Multiply(x=w440, y="Bv_y") -> (x*y=w439:fxp<+/-,55,16>)
        n228 = Add(x=w442, y=w439) -> (x+y=w438:fxp<+/-,55,16>)
      }
    }
    "Fr_y" <- w434
  }
  n229 = while "Command type" {
    stop <- FALSE stop-if-true
    n230 = case shown="1" "Command_y" {
      tunnel: ["Dyr_step" w454] -> w449
      frame 0, Default {
        # "Step"
      }
      frame 1 {
        # "Sine"
        n231 = local read "Dyr_sin"() -> (w454:fxp<+/-,22,7>)
      }
    }
    "Dyr_for" <- w449
    n232 = case shown="0, Default" "Command_p" {
      tunnel: ["Dpr_step" w452] -> w447
      frame 0, Default {
        # "Step"
      }
      frame 1 {
        # "Sine"
        n233 = local read "Dpr_sin"() -> (w452:fxp<+/-,22,7>)
      }
    }
    "Dpr_for" <- w447
  }
  n234 = while "Sine wave gene" {
    stop <- FALSE stop-if-true
    w460 = fxp<+,20,3> 6.2831878662109375  # 2*pi
    w492 = fxp<+,20,3> 6.2831878662109375  # 2*pi
    n235 = local read "Time now(s)"() -> (w498:fxp<+,52,14>)
    n236 = local read "Sin wave freq._y (Hz)"() -> (w491:fxp<+/-,32,6>)
    n237 = Multiply(x="Sin wave freq._y (Hz)", y=fxp<+/-,10,3> 2.0) -> (x*y=w499:fxp<+/-,41,9>)
    n238 = local read "Sin magnitude_y"() -> (w489:fxp<+/-,21,6>)
    n239 = local read "Sin magnitude_y"() -> (w482:fxp<+/-,21,6>)
    n240 = local read "Sin omega_y"() -> (w485:fxp<+/-,34,9>)
    n241 = Multiply(x=w499, y=w498) -> (x*y=w497:fxp<+/-,41,19>)
    n242 = Square(x=w485) -> (x^2=w484:fxp<+,34,18>)
    n243 = xnode "High Throughput Sine & Cosine"("x (pi)"=w497) -> ("sin(x)"=w479:fxp<+/-,16,2>, "cos(x)"=w487:fxp<+/-,16,2>)
    n244 = Multiply(x=w492, y=w491) -> (x*y=w490:fxp<+/-,34,9>)
    "Sin omega_y" <- w490
    n245 = Negate(x=w484) -> (-x=w483:fxp<+/-,35,19>)
    n246 = Multiply(x=w490, y=w489) -> (x*y=w488:fxp<+/-,33,15>)
    n247 = Multiply(x=w483, y=w482) -> (x*y=w481:fxp<+/-,34,20>)
    n248 = Multiply(x=w487, y=w488) -> (x*y=→"Dyr_sin_d":fxp<+/-,33,15>)
    n249 = Multiply(x="Sin magnitude_y", y=w479) -> (x*y=w495:fxp<+/-,37,8>)
    n250 = Multiply(x=w479, y=w481) -> (x*y=→"Dyr_sin_dd":fxp<+/-,35,20>)
    n251 = Add(x=w495, y="Sin offset_y") -> (x+y=→"Dyr_sin":fxp<+/-,37,8>)
    n252 = local read "Sin wave freq._p (Hz)"() -> (w456:fxp<+/-,32,6>)
    n253 = local read "Time now(s)"() -> (w474:fxp<+,52,14>)
    n254 = local read "Sin magnitude_p"() -> (w457:fxp<+/-,21,6>)
    n255 = local read "Sin magnitude_p"() -> (w459:fxp<+/-,21,6>)
    n256 = local read "Sin omega_p"() -> (w458:fxp<+/-,34,9>)
    n257 = Multiply(x="Sin wave freq._p (Hz)", y=fxp<+/-,10,3> 2.0) -> (x*y=w478:fxp<+/-,42,9>)
    n258 = Multiply(x=w478, y=w474) -> (x*y=w475:fxp<+/-,41,19>)
    n259 = Square(x=w458) -> (x^2=w470:fxp<+,34,18>)
    n260 = xnode "High Throughput Sine & Cosine"("x (pi)"=w475) -> ("sin(x)"=w461:fxp<+/-,16,2>, "cos(x)"=w466:fxp<+/-,16,2>)
    n261 = Multiply(x=w460, y=w456) -> (x*y=w473:fxp<+/-,34,9>)
    "Sin omega_p" <- w473
    n262 = Negate(x=w470) -> (-x=w469:fxp<+/-,35,19>)
    n263 = Multiply(x=w473, y=w457) -> (x*y=w472:fxp<+/-,33,15>)
    n264 = Multiply(x=w469, y=w459) -> (x*y=w468:fxp<+/-,35,19>)
    n265 = Multiply(x=w466, y=w472) -> (x*y=→"Dpr_sin_d":fxp<+/-,33,15>)
    n266 = Multiply(x=w461, y=w468) -> (x*y=→"Dpr_sin_dd":fxp<+/-,35,20>)
    n267 = Multiply(x="Sin magnitude_p", y=w461) -> (x*y=w464:fxp<+/-,37,8>)
    n268 = Add(x=w464, y="Sin offset_p") -> (x+y=→"Dpr_sin":fxp<+/-,37,8>)
  }
  n269 = while "Time reset" {
    shift-right: [w571] -> _
    shift-left: _ -> [w572]
    shift-right: [w566] -> _
    shift-left: _ -> [w567]
    stop <- FALSE stop-if-true
    n270 = local read "Stop motor_y"() -> (w573:bool)
    n271 = call "Tick Count3"() -> ("Tick Count(uSec)"=w571:u32)
    n272 = Subtract(x=w571, y=w572) -> (x-y=w570:u32)
    n273 = Add(x=w567, y=w570) -> (x+y=w569:u32)
    n274 = Select(t=u32 0, s=w573, f=w569) -> (s? t:f=w566:u32)
    n275 = To Fixed-Point(number=w566) -> (fixed-point=w565:fxp<+,32,32>)  [unwired: 1 in]
    n276 = Multiply(x=fxp<+,20,-18> 1.0000003385357559e-06, y=w565) -> (x*y=→"Time now(s)":fxp<+,52,14>)
  }
  n277 = while "Ini" {
    stop <- FALSE stop-if-true
    n278 = case shown="True" "Ini coe." {
      frame False {
      }
      frame True {
        w583 = T2 20 items=["50.000 kS/s (NI 9237)"=1, "25.000 kS/s (NI 9237)"=2, "16.667 kS/s (NI 9237)"=3, "12.500 kS/s (NI 9237)"=4, "10.000 kS/s (NI 9237)"=5, "8.333 kS/s (NI 9237)"=6, "7.143 kS/s (NI 9237)"=7, "6.250 kS/s (NI 9237)"=8, "5.556 kS/s (NI 9237)"=9, "5.000 kS/s (NI 9237)"=10, "4.545 kS/s (NI 9237)"=11, "4.167 kS/s (NI 9237)"=12, "3.846 kS/s (NI 9237)"=13, "3.571 kS/s (NI 9237)"=14, "3.333 kS/s (NI 9237)"=15, "3.125 kS/s (NI 9237)"=16, "2.941 kS/s (NI 9237)"=17, "2.778 kS/s (NI 9237)"=18, "2.632 kS/s (NI 9237)"=19, "2.500 kS/s (NI 9237)"=20, "2.381 kS/s (NI 9237)"=21, "2.273 kS/s (NI 9237)"=22, "2.174 kS/s (NI 9237)"=23, "2.083 kS/s (NI 9237)"=24, "2.000 kS/s (NI 9237)"=25, "1.923 kS/s (NI 9237)"=26, "1.852 kS/s (NI 9237)"=27, "1.786 kS/s (NI 9237)"=28, "1.724 kS/s (NI 9237)"=29, "1.667 kS/s (NI 9237)"=30, "1.613 kS/s (NI 9237)"=31] ("Data Rate")
        w600 = i16 0 items=["Step", "Sine"] ("Command_p")
        w601 = i16 2 items=["Raw", "Avg.", "Avg. w. filter"] ("Strain selection_p")
        w602 = i16 0 items=["Step", "Sine"] ("Command_y")
        w603 = i16 2 items=["Raw", "Avg.", "Avg. w. filter"] ("Strain selection_y")
        w605 = fxp<+/-,25,-10> 5.851034075021744e-07  # S/F coeff_p
        w604 = fxp<+/-,25,-10> 1.0477961041033268e-06  # S/F coeff_y
        w611 = i16 0 items=["Backward", "Forward"] ("Drive mode")
        n279 = local write "Sin wave freq._y (Hz)"(fxp<+/-,32,6> 1.0 ("Sin wave freq. (Hz)")) -> ()
        n280 = local write "Sin magnitude_y"(fxp<+/-,22,7> 5.0 ("Sin magnitude")) -> ()
        n281 = local write "fy_tolorance"(fxp<+,22,6> 5.0 ("f_tolorance")) -> ()
        n282 = local write "Sin offset_y"(fxp<+/-,38,9> 0.0 ("Sin offset")) -> ()
        n283 = local write "Dyr_step"(fxp<+/-,22,7> 0.0 ("Dr")) -> ()
        n284 = local write "Kp_y"(fxp<+/-,36,9> 30.0 ("Kp")) -> ()
        n285 = local write "Kd_y"(fxp<+/-,36,9> 0.0 ("Kd")) -> ()
        n286 = local write "Kv_y"(fxp<+/-,22,8> 0.0 ("Kv")) -> ()
        n287 = local write "Bv_y"(fxp<+/-,22,8> 0.0 ("Bv")) -> ()
        n288 = local write "Ki_y"(fxp<+/-,36,9> 0.0 ("Ki")) -> ()
        n289 = local write "S/F coeff_p"(w605) -> ()
        n290 = local write "S/F coeff_y"(w604) -> ()
        n291 = local write "Data Rate"(w583) -> ()
        n292 = local write "dFy_add"(FALSE ("dF_add")) -> ()
        n293 = local write "dFp_add"(FALSE ("dFp_add")) -> ()
        n294 = local write "Sin wave freq._p (Hz)"(fxp<+/-,32,6> 1.0 ("Sin wave freq._p (Hz)")) -> ()
        n295 = local write "Sin magnitude_p"(fxp<+/-,21,6> 5.0 ("Sin magnitude_p")) -> ()
        n296 = local write "fp_tolorance"(fxp<+,22,6> 5.0 ("fp_tolorance")) -> ()
        n297 = local write "Sin offset_p"(fxp<+/-,22,7> 0.0 ("Sin offset_p")) -> ()
        n298 = local write "Dpr_step"(fxp<+/-,22,7> 0.0 ("Dpr_step")) -> ()
        n299 = local write "Kp_p"(fxp<+/-,36,9> 30.0 ("Kp_p")) -> ()
        n300 = local write "Kd_p"(fxp<+/-,36,9> 0.0 ("Kd_p")) -> ()
        n301 = local write "Kv_p"(fxp<+/-,22,8> 0.0 ("Kv_p")) -> ()
        n302 = local write "Bv_p"(fxp<+/-,22,8> 0.0 ("Bv_p")) -> ()
        n303 = local write "Ki_p"(fxp<+/-,36,9> 0.0 ("Ki_p")) -> ()
        n304 = local write "Strain selection_p"(w601) -> ()
        n305 = local write "Strain selection_y"(w603) -> ()
        n306 = local write "Command_p"(w600) -> ()
        n307 = local write "Command_y"(w602) -> ()
        n308 = local write "Drive mode"(w611) -> ()
        n309 = local write "Dp_d_M_avg_Tc (uSec)"(u32 1000 ("D_d_M_avg_Tc (uSec)")) -> ()
        n310 = local write "Dy_d_M_avg_Tc (uSec)"(1000 ("Dy_d_M_avg_Tc (uSec)")) -> ()
        n311 = local write "Mag. factor_p"(fxp<+/-,20,3> 1.0 ("Mag. factor_p")) -> ()
        n312 = local write "Mag. factor_y"(fxp<+/-,20,3> 1.0 ("Mag. factor_y")) -> ()
        n313 = local write "Belt_out_p"(fxp<+/-,7,7> 36.0 ("Belt_op")) -> ()
        n314 = local write "Belt_out_y"(fxp<+/-,7,7> 36.0 ("Belt_oy")) -> ()
        n315 = local write "Belt_in_p"(fxp<+/-,6,6> 16.0 ("Belt_mp")) -> ()
        n316 = local write "Belt_in_y"(fxp<+/-,6,6> 16.0 ("Belt_my")) -> ()
        n317 = local write "mt0_p1"(u32 628319 ("mt0_p1")) -> ()
        n318 = local write "mt0_p2"(u32 628319 ("mt0_p2")) -> ()
        n319 = local write "mt0_y1"(u32 628319 ("mt0_y1")) -> ()
        n320 = local write "mt0_y2"(u32 628319 ("mt0_y2")) -> ()
      }
    }
  }
  n321 = while "FIFO" {
    stop <- FALSE stop-if-true
    n322 = flat-sequence {
      frame #0 {
        n323 = call "Loop Timer"("Count(uSec)"=u32 1000) -> ()  [unwired: 1 out]
      }
      frame #1 {
        # "imp ctrl"
        n324 = local read "D_y(mm)"() -> (w637:fxp<+/-,32,7>)
        n325 = local read "Raw Strain_y"() -> (w636:fxp<+/-,36,4>)
        n326 = local read "Strain_y (Avg8 w. f)"() -> (w635:fxp<+/-,36,8>)
        n327 = local read "Force_y"() -> (w634:fxp<+/-,32,10>)
        n328 = local read "D_y1"() -> (w630:fxp<+/-,32,7>)
        n329 = local read "D_y2"() -> (w631:fxp<+/-,32,7>)
        n330 = local read "omega_y1 (T)"() -> (w632:fxp<+/-,36,13>)
        n331 = local read "omega_y2 (Mavg)"() -> (w620:fxp<+/-,36,14>)
        n332 = local read "D_p(mm)"() -> (w629:fxp<+/-,32,7>)
        n333 = local read "Raw Strain_p"() -> (w628:fxp<+/-,36,4>)
        n334 = local read "Strain_p (Avg8 w. f)"() -> (w627:fxp<+/-,36,8>)
        n335 = local read "Force_p"() -> (w626:fxp<+/-,32,10>)
        n336 = local read "D_p1"() -> (w625:fxp<+/-,32,7>)
        n337 = local read "D_p2"() -> (w624:fxp<+/-,32,7>)
        n338 = local read "omega_p1 (T)"() -> (w623:fxp<+/-,36,13>)
        n339 = local read "omega_p2 (Mavg)"() -> (w622:fxp<+/-,36,14>)
        n340 = Build Array(w637, w636, w635, w634, w630, w631, w632, w620, w629, w628, w627, w626, w625, w624, w623, w622) -> (w621:fxp<+/-,46,14>[])
        n341 = xnode ("FIFO Write")("Element"=w621, "Timeout"=0) -> ()  [unwired: 1 in, 2 out]
      }
    }
  }
  n342 = while "PID force controller_y" {
    stop <- FALSE stop-if-true
    n343 = local read "Force_y"() -> (w639:fxp<+/-,32,10>)
    n344 = local read "fyt_d"() -> (w648:fxp<+/-,36,18>)
    n345 = local read "Fr_y"() -> (w640:fxp<+/-,32,10>)
    n346 = Subtract(x=w640, y=w639) -> (x-y=w638:fxp<+/-,33,11>)
    "fy_tilde" <- w638
    n347 = Absolute Value(x=w638) -> (abs(x)=w655:fxp<+,32,10>)
    n348 = local read "fyt_i"() -> (w644:fxp<+/-,36,16>)
    n349 = Multiply(x="Kp_y", y=w638) -> (x*y=w646:fxp<+/-,64,23>)
    n350 = Multiply(x="Kd_y", y=w648) -> (x*y=w647:fxp<+/-,64,27>)
    n351 = Multiply(x="Ki_y", y=w644) -> (x*y=w642:fxp<+/-,64,25>)
    n352 = Add(x=w646, y=w647) -> (x+y=w643:fxp<+/-,64,28>)
    n353 = Greater?(x=w655, y="fy_tolorance") -> (0:w653:bool)
    n354 = Add(x=w643, y=w642) -> (x+y=w641:fxp<+/-,64,29>)
    n355 = Select(t=w641, s=w653, f=fxp<+/-,51,14> 0.0) -> (s? t:f=→"Fy_PID":fxp<+/-,64,29>)
  }
  n356 = for {
    N: w2 -> [_]
    tunnel: [w658] -> w4 mode=indexing
    tunnel: [w657] -> w3 mode=indexing
    tunnel: [w657] -> w1
    n357 = local read "Dp_d_M_avg_Tc (uSec)"() -> (w657:i32)
    n358 = local read "Encoder Position_p2"() -> (w658:i32)
    n359 = call "Wait5"("Count(uSec)"=w657) -> ()  [unwired: 1 out]
  }
  n360 = while {
    tunnel: w24 -> [w703]
    tunnel: [w677] -> w17
    shift-right: [w701] -> _
    shift-left: _ -> [w702]
    shift-right: [w697] -> _
    shift-left: _ -> [w698]
    shift-right: [w692] -> _
    shift-left: _ -> [w691]
    shift-right: [w691] -> _
    shift-left: _ -> [w690]
    shift-right: [w690] -> _
    shift-left: _ -> [w689]
    shift-right: [w689] -> _
    shift-left: _ -> [w688]
    shift-right: [w688] -> _
    shift-left: _ -> [w687]
    shift-right: [w687] -> _
    shift-left: _ -> [w686]
    shift-right: [w686] -> _
    shift-left: _ -> [w685]
    tunnel: w24 -> [w681]
    shift-right: [w674] -> _
    shift-left: _ -> [w675]
    shift-right: [w670] -> _
    shift-left: _ -> [w669]
    shift-right: [w669] -> _
    shift-left: _ -> [w668]
    shift-right: [w668] -> _
    shift-left: _ -> [w667]
    shift-right: [w667] -> _
    shift-left: _ -> [w666]
    shift-right: [w666] -> _
    shift-left: _ -> [w665]
    shift-right: [w665] -> _
    shift-left: _ -> [w664]
    shift-right: [w664] -> _
    shift-left: _ -> [w663]
    stop <- w678 stop-if-true
    w672 = fxp<+,20,2> 2.115001678466797  # Gage Factor
    n361 = xnode "FPGA I/O Node"("error in"=w703) -> ("error out"=w677:errorcluster, "Mod6/AI2"=w699:fxp<+/-,24,-4>)  [unwired: 1 in, 1 out]
    n362 = xnode "FPGA I/O Node"("error in"=w681) -> ("error out"=w679:errorcluster, "Mod6/AI3"=w673:fxp<+/-,24,-4>)  [unwired: 1 in, 1 out]
    n363 = Or(x=w677, y="Stop (Strain)") -> (x .or. y?=w680:bool)
    n364 = Select(t=w673, s="Strain gage reset_p", f=w675) -> (s? t:f=w674:fxp<+/-,24,-4>)
    n365 = Select(t=w699, s="Strain gage reset_y", f=w702) -> (s? t:f=w701:fxp<+/-,24,-4>)
    n366 = Or(x=w680, y=w679) -> (x .or. y?=w678:bool)
    n367 = Subtract(x=w673, y=w674) -> (x-y=w671:fxp<+/-,30,-3>)
    "Mod6/AI3" <- w671
    n368 = Subtract(x=w699, y=w701) -> (x-y=w700:fxp<+/-,30,-3>)
    "Mod6/AI2" <- w700
    n369 = Multiply(x=w672, y=w700) -> (x*y=w692:fxp<+/-,41,6>)
    "Raw Strain_y" <- w692
    n370 = Multiply(x=w672, y=w671) -> (x*y=w670:fxp<+/-,50,-1>)
    "Raw Strain_p" <- w670
    n371 = call "average_v2.vi"("Numeric 8"=w663, "Numeric"=w670, "Numeric 7"=w664, "Numeric 2"=w669, "Numeric 6"=w665, "Numeric 5"=w666, "Numeric 4"=w667, "Numeric 3"=w668) -> ("Mean (8pt)"=w662:fxp<+/-,32,4>)  [unwired: 1 in, 2 out]
    "Strain_p (Avg8)" <- w662
    n372 = call "average_v2.vi"("Numeric 8"=w685, "Numeric"=w692, "Numeric 7"=w686, "Numeric 2"=w691, "Numeric 6"=w687, "Numeric 5"=w688, "Numeric 4"=w689, "Numeric 3"=w690) -> ("Mean (8pt)"=w684:fxp<+/-,32,4>)  [unwired: 1 in, 2 out]
    "Strain_y (Avg8)" <- w684
    n373 = call "Tick Count"() -> ("Tick Count(uSec)"=w697:u32)
    n374 = xnode "Butterworth Filter"("input data"=w662, "scaled coefficients"="Strain_p Avg.8 coeff.") -> ("output data"=→"Strain_p (Avg8 w. f)":fxp<+/-,36,8>)  [unwired: 1 in]
    n375 = xnode "Butterworth Filter"("input data"=w684, "scaled coefficients"="Strain_y Avg8 coeff.") -> ("output data"=→"Strain_y (Avg8 w. f)":fxp<+/-,32,4>)  [unwired: 1 in]
    n376 = Subtract(x=w697, y=w698) -> (x-y=w695:fxp<+/-,32,16>)
    n377 = Divide(x=fxp<+,7,10> 1000.0, y=w695) -> (x/y=→"Loop rate (kHz)":fxp<+/-,40,27>)
  }
  n378 = for {
    N: w5 -> [_]
    tunnel: [w722] -> w8 mode=indexing
    tunnel: [w721] -> w7 mode=indexing
    tunnel: [w720] -> w6
    n379 = local read "Dy_d_M_avg_Tc (uSec)"() -> (w720:i32)
    n380 = local read "Encoder Position_y2"() -> (w722:i32)
    n381 = call "Wait4"("Count(uSec)"=w720) -> ("Tick Count(uSec)"=w721:u32)
  }
  n382 = for {
    N: w13 -> [_]
    tunnel: [w725] -> w12 mode=indexing
    tunnel: [w724] -> w11 mode=indexing
    tunnel: ["Dy_d_M_avg_Tc (uSec)"] -> w10
    n383 = local read "Encoder Position_y1"() -> (w724:i32)
    n384 = call "Wait3"("Count(uSec)"="Dy_d_M_avg_Tc (uSec)") -> ("Tick Count(uSec)"=w725:u32)
  }
  n385 = for {
    N: w16 -> [_]
    tunnel: ["Dp_d_M_avg_Tc (uSec)"] -> w9
    tunnel: [w727] -> w15 mode=indexing
    tunnel: [w726] -> w14 mode=indexing
    n386 = local read "Encoder Position_p1"() -> (w726:i32)
    n387 = call "Wait2"("Count(uSec)"="Dp_d_M_avg_Tc (uSec)") -> ("Tick Count(uSec)"=w727:u32)
  }
  n388 = while "Omega_p2 (Mavg)" {
    shift-right: [w730] -> _
    shift-left: w4 -> [w751]
    shift-right: [w731] -> _
    shift-left: w3 -> [w749]
    shift-right: [w735] -> _
    shift-left: _ -> [w733]
    tunnel: w2 -> [w747]
    tunnel: w1 -> [w752]
    stop <- FALSE stop-if-true
    w736 = fxp<+/-,27,3> 3.1415926814079285  # pi
    w739 = fxp<+,32,0> 0.1953125  # 800/4096
    w744 = fxp<+/-,32,0> 0.3183098859153688  # L/2/pi
    n389 = call "Tick Count9"() -> ("Tick Count(uSec)"=w746:u32)
    n390 = Index Array(array=w749, index=0) -> (element=w748:i32)
    n391 = Index Array(array=w751, index=0) -> (element=w750:i32)
    n392 = Multiply(x=w747, y=w752) -> (x*y=w755:i32)
    n393 = Add(x=w755, y=w748) -> (x+y=w754:i32)
    n394 = Greater Or Equal?(x=w746, y=w754) -> (x >= y?=w753:bool)
    n395 = case shown="True" w753 {
      tunnel: w751 -> [w759 w774]
      tunnel: w750 -> [_ w766]
      tunnel: w749 -> [w760 w775]
      tunnel: w748 -> [_ w776]
      tunnel: w747 -> [_ w773]
      tunnel: w746 -> [_ w761]
      tunnel: [w759 w764] -> w730
      tunnel: [w760 w763] -> w731
      tunnel: [w758 w762] -> w735
      tunnel: w733 -> [w758 _]
      frame False {
      }
      frame True {
        n396 = local read "Encoder Position_p2"() -> (w765:i32)
        n397 = Subtract(x=w761, y=w776) -> (x-y=w777:u32)
        n398 = Insert Into Array(array=w775, new element=w761) -> (w779:i32[])  [unwired: 1 in]
        n399 = Subtract(x=w765, y=w766) -> (x-y=w770:i32)
        n400 = Insert Into Array(array=w774, index=w773, new element=w765) -> (w780:i32[])
        n401 = To Fixed-Point(number=w777) -> (fixed-point=w767:fxp<+,32,32>)  [unwired: 1 in]
        n402 = Multiply(x=w770, y=2500) -> (x*y=w771:i32)
        n403 = To Fixed-Point(number=w771) -> (fixed-point=w772:fxp<+/-,32,32>)  [unwired: 1 in]
        n404 = Delete From Array(array=w779, length=1, index=0) -> (array with subset deleted=w763:i32[])  [unwired: 1 out]
        n405 = Delete From Array(array=w780, length=1, index=0) -> (array with subset deleted=w764:i32[])  [unwired: 1 out]
        n406 = Divide(x=w772, y=w767) -> (x/y=w762:fxp<+/-,64,32>)
      }
    }
    n407 = local read "Mag. factor_p"() -> (w738:fxp<+/-,20,3>)
    n408 = local read "Belt_in_p"() -> (w741:fxp<+/-,6,6>)
    n409 = local read "Belt_out_p"() -> (w740:fxp<+/-,7,7>)
    n410 = Divide(x=w739, y=w738) -> (x/y=w729:fxp<+/-,32,1>)
    n411 = Multiply(x=w736, y=w735) -> (x*y=w737:fxp<+/-,64,35>)
    n412 = Multiply(x=w744, y=w741) -> (x*y=w745:fxp<+/-,38,6>)
    n413 = Multiply(x=w729, y=w737) -> (x*y=w732:fxp<+/-,64,36>)
    "omega_p2 (Mavg)" <- w732
    n414 = Divide(x=w745, y=w740) -> (x/y=w743:fxp<+/-,45,6>)
    n415 = Multiply(x=w743, y=w732) -> (x*y=→"Dp2_d (Mavg)":fxp<+/-,64,41>)
  }
  n416 = while "Omega_y1 (Mavg)" {
    tunnel: w13 -> [w801]
    shift-right: [w799] -> _
    shift-left: w12 -> [w804]
    shift-right: [w798] -> _
    shift-left: w11 -> [w800]
    shift-right: [w793] -> _
    shift-left: _ -> [w797]
    tunnel: w10 -> [w792]
    stop <- FALSE stop-if-true
    w786 = fxp<+/-,32,0> 0.3183098859153688  # L/2/pi
    w795 = fxp<+/-,27,3> 0.007853984832763672  # 2*pi/800
    n417 = call "Tick Count6"() -> ("Tick Count(uSec)"=w805:u32)
    n418 = Index Array(array=w804, index=0) -> (element=w803:u32)
    n419 = Index Array(array=w800, index=0) -> (element=w802:i32)
    n420 = Multiply(x=w801, y=w792) -> (x*y=w807:i32)
    n421 = Add(x=w807, y=w803) -> (x+y=w806:u32)
    n422 = Greater Or Equal?(x=w805, y=w806) -> (x >= y?=w796:bool)
    n423 = case shown="True" w796 {
      tunnel: w805 -> [_ w828]
      tunnel: w801 -> [_ w825]
      tunnel: w804 -> [w812 w827]
      tunnel: w803 -> [_ w826]
      tunnel: w802 -> [_ w822]
      tunnel: w800 -> [w811 w824]
      tunnel: [w810 w820] -> w793
      tunnel: [w812 w819] -> w799
      tunnel: [w811 w818] -> w798
      tunnel: w797 -> [w810 _]
      frame False {
      }
      frame True {
        # "count/s"
        n424 = local read "Encoder Position_y1"() -> (w821:i32)
        n425 = Subtract(x=w828, y=w826) -> (x-y=w829:u32)
        n426 = Insert Into Array(array=w827, new element=w828) -> (w831:u32[])  [unwired: 1 in]
        n427 = Subtract(x=w821, y=w822) -> (x-y=w816:i32)
        n428 = Insert Into Array(array=w824, index=w825, new element=w821) -> (w832:i32[])
        n429 = To Fixed-Point(number=w829) -> (fixed-point=w815:fxp<+,32,32>)  [unwired: 1 in]
        n430 = To Fixed-Point(number=w816) -> (fixed-point=w823:fxp<+/-,32,32>)  [unwired: 1 in]
        n431 = Divide(x=w815, y=fxp<+,32,32> 1000000.0) -> (x/y=w814:fxp<+/-,64,32>)
        n432 = Delete From Array(array=w831, length=1, index=0) -> (array with subset deleted=w819:u32[])  [unwired: 1 out]
        n433 = Delete From Array(array=w832, length=1, index=0) -> (array with subset deleted=w818:i32[])  [unwired: 1 out]
        n434 = Divide(x=w823, y=w814) -> (x/y=w820:fxp<+/-,64,65>)
      }
    }
    n435 = local read "Belt_in_y"() -> (w788:fxp<+/-,6,6>)
    n436 = Multiply(x=w795, y=w793) -> (x*y=w791:fxp<+/-,64,68>)
    n437 = local read "Belt_out_y"() -> (w789:fxp<+/-,7,7>)
    n438 = Multiply(x=w786, y=w788) -> (x*y=w787:fxp<+/-,38,6>)
    n439 = Multiply(x=fxp<+/-,2,2> 1.0 ("f"), y=w791) -> (x*y=w790:fxp<+/-,64,70>)
    "omega_y1 (Mavg)" <- w790
    n440 = Divide(x=w787, y=w789) -> (x/y=w785:fxp<+/-,45,6>)
    n441 = Multiply(x=w785, y=w790) -> (x*y=→"Dy1_d (Mavg)":fxp<+/-,64,75>)
  }
  n442 = while "Omega_p1 (Mavg)" {
    tunnel: w16 -> [w853]
    shift-right: [w851] -> _
    shift-left: w15 -> [w856]
    shift-right: [w850] -> _
    shift-left: w14 -> [w852]
    shift-right: [w849] -> _
    shift-left: _ -> [w848]
    tunnel: w9 -> [w846]
    stop <- FALSE stop-if-true
    w840 = fxp<+/-,27,3> 3.1415926814079285  # pi
    w839 = fxp<+/-,32,0> 0.3183098859153688  # L/2/pi
    n443 = call "Tick Count5"() -> ("Tick Count(uSec)"=w857:u32)
    n444 = Index Array(array=w856, index=0) -> (element=w855:u32)
    n445 = Index Array(array=w852, index=0) -> (element=w854:i32)
    n446 = Multiply(x=w853, y=w846) -> (x*y=w859:i32)
    n447 = Add(x=w859, y=w855) -> (x+y=w858:u32)
    n448 = Greater Or Equal?(x=w857, y=w858) -> (x >= y?=w847:bool)
    n449 = case shown="True" w847 {
      tunnel: w857 -> [_ w880]
      tunnel: w853 -> [_ w877]
      tunnel: w856 -> [w864 w879]
      tunnel: w855 -> [_ w878]
      tunnel: w854 -> [_ w874]
      tunnel: w852 -> [w863 w876]
      tunnel: [w862 w872] -> w849
      tunnel: [w864 w871] -> w851
      tunnel: [w863 w870] -> w850
      tunnel: w848 -> [w862 _]
      frame False {
      }
      frame True {
        n450 = local read "Encoder Position_p1"() -> (w873:i32)
        n451 = Subtract(x=w880, y=w878) -> (x-y=w881:u32)
        n452 = Subtract(x=w873, y=w874) -> (x-y=w866:i32)
        n453 = Insert Into Array(array=w879, new element=w880) -> (w883:u32[])  [unwired: 1 in]
        n454 = Insert Into Array(array=w876, index=w877, new element=w873) -> (w884:i32[])
        n455 = To Fixed-Point(number=w881) -> (fixed-point=w868:fxp<+,32,32>)  [unwired: 1 in]
        n456 = Multiply(x=w866, y=2500) -> (x*y=w867:i32)
        n457 = To Fixed-Point(number=w867) -> (fixed-point=w875:fxp<+/-,32,32>)  [unwired: 1 in]
        n458 = Delete From Array(array=w883, length=1, index=0) -> (array with subset deleted=w871:u32[])  [unwired: 1 out]
        n459 = Delete From Array(array=w884, length=1, index=0) -> (array with subset deleted=w870:i32[])  [unwired: 1 out]
        n460 = Divide(x=w875, y=w868) -> (x/y=w872:fxp<+/-,64,32>)
      }
    }
    n461 = local read "Belt_in_p"() -> (w844:fxp<+/-,6,6>)
    n462 = local read "Belt_out_p"() -> (w843:fxp<+/-,7,7>)
    n463 = Multiply(x=w840, y=w849) -> (x*y=w845:fxp<+/-,64,35>)
    n464 = Multiply(x=w839, y=w844) -> (x*y=w842:fxp<+/-,38,6>)
    n465 = Multiply(x=fxp<+/-,2,2> 1.0 ("f"), y=w845) -> (x*y=w838:fxp<+/-,64,37>)
    "omega_p1 (Mavg)" <- w838
    n466 = Divide(x=w842, y=w843) -> (x/y=w837:fxp<+/-,45,6>)
    n467 = Multiply(x=w837, y=w838) -> (x*y=→"Dp1_d (Mavg)":fxp<+/-,64,42>)
  }
  n468 = while "Omega_y2 (Mavg)" {
    shift-right: [w889] -> _
    shift-left: w7 -> [w909]
    shift-right: [w888] -> _
    shift-left: w8 -> [w911]
    tunnel: w6 -> [w907]
    tunnel: w5 -> [w905]
    shift-right: [w892] -> _
    shift-left: _ -> [w903]
    stop <- FALSE stop-if-true
    w894 = fxp<+/-,27,3> 0.007853984832763672  # 2*pi/800
    w896 = fxp<+,32,0> 0.1953125  # 800/4096
    w901 = fxp<+/-,32,0> 0.3183098859153688  # L/2/pi
    n469 = call "Tick Count8"() -> ("Tick Count(uSec)"=w910:u32)
    n470 = Index Array(array=w909, index=0) -> (element=w908:u32)
    n471 = Index Array(array=w911, index=0) -> (element=w906:i32)
    n472 = Multiply(x=w905, y=w907) -> (x*y=w913:i32)
    n473 = Add(x=w913, y=w908) -> (x+y=w912:u32)
    n474 = Greater Or Equal?(x=w910, y=w912) -> (x >= y?=w904:bool)
    n475 = case shown="True" w904 {
      tunnel: w911 -> [w916 w929]
      tunnel: w910 -> [_ w932]
      tunnel: w909 -> [w917 w931]
      tunnel: w908 -> [_ w930]
      tunnel: w906 -> [_ w919]
      tunnel: w905 -> [_ w928]
      tunnel: [w917 w927] -> w889
      tunnel: [w916 w926] -> w888
      tunnel: [w918 w921] -> w892
      tunnel: w903 -> [w918 _]
      frame False {
      }
      frame True {
        n476 = local read "Encoder Position_y2"() -> (w920:i32)
        n477 = Subtract(x=w932, y=w930) -> (x-y=w935:u32)
        n478 = Insert Into Array(array=w931, new element=w932) -> (w937:u32[])  [unwired: 1 in]
        n479 = Insert Into Array(array=w929, index=w928, new element=w920) -> (w938:i32[])
        n480 = Subtract(x=w920, y=w919) -> (x-y=w924:i32)
        n481 = To Fixed-Point(number=w935) -> (fixed-point=w934:fxp<+,32,32>)  [unwired: 1 in]
        n482 = To Fixed-Point(number=w924) -> (fixed-point=w925:fxp<+/-,32,32>)  [unwired: 1 in]
        n483 = Divide(x=w934, y=fxp<+,32,32> 1000000.0) -> (x/y=w923:fxp<+/-,64,32>)
        n484 = Delete From Array(array=w937, length=1, index=0) -> (array with subset deleted=w927:u32[])  [unwired: 1 out]
        n485 = Delete From Array(array=w938, length=1, index=0) -> (array with subset deleted=w926:i32[])  [unwired: 1 out]
        n486 = Divide(x=w925, y=w923) -> (x/y=w921:fxp<+/-,64,65>)
      }
    }
    n487 = local read "Mag. factor_y"() -> (w895:fxp<+/-,20,3>)
    n488 = local read "Belt_in_y"() -> (w898:fxp<+/-,6,6>)
    n489 = local read "Belt_out_y"() -> (w897:fxp<+/-,7,7>)
    n490 = Multiply(x=w894, y=w892) -> (x*y=w893:fxp<+/-,64,68>)
    n491 = Divide(x=w896, y=w895) -> (x/y=w887:fxp<+/-,32,1>)
    n492 = Multiply(x=w901, y=w898) -> (x*y=w902:fxp<+/-,38,6>)
    n493 = Multiply(x=w887, y=w893) -> (x*y=w890:fxp<+/-,64,69>)
    "omega_y2 (Mavg)" <- w890
    n494 = Divide(x=w902, y=w897) -> (x/y=w900:fxp<+/-,45,6>)
    n495 = Multiply(x=w900, y=w890) -> (x*y=→"Dy2_d (Mavg)":fxp<+/-,64,74>)
  }
  n496 = while "Quadrature drive_p" {
    stop <- FALSE stop-if-true
    n497 = local read "Drive mode"() -> (w942:i16)
    n498 = case shown="1" w942 {
      tunnel: [w952 w953] -> w941
      frame 0, Default {
        # "Backward"
        n499 = local read "Fp_PID"() -> (w952:fxp<+/-,36,16>)
      }
      frame 1 {
        # "Forward"
        n500 = local read "Fr_p"() -> (w953:fxp<+/-,32,10>)
      }
    }
    n501 = local read "dFp_PID"() -> (w945:fxp<+/-,36,18>)
    n502 = local read "omega_p (rad/s)"() -> (w949:fxp<+/-,36,13>)
    n503 = Select(t=w945, s="dFp_add", f=fxp<+,1,1> 0.0) -> (s? t:f=w948:fxp<+/-,36,18>)
    n504 = call "Oriental_step_motor_PKP225.vi"("F_Threshold"="F_Threshold_p", "dFmr"=w948, "omega"=w949, "Fmr"=w941) -> ("vq_F"=→"vq_p_F":fxp<+/-,36,9>, "vd_F"=→"vd_p_F":fxp<+/-,36,9>)  [unwired: 6 in]
  }
  n505 = while "PID force controller_p" {
    shift-right: [w958] -> _
    shift-left: _ -> [w957]
    stop <- FALSE stop-if-true
    n506 = local read "Force_p"() -> (w970:fxp<+/-,32,10>)
    n507 = local read "fpt_d"() -> (w966:fxp<+/-,36,18>)
    n508 = local read "Fr_p"() -> (w971:fxp<+/-,32,10>)
    n509 = Subtract(x=w971, y=w970) -> (x-y=w968:fxp<+/-,33,11>)
    "fp_tilde" <- w968
    n510 = local read "fpt_i"() -> (w962:fxp<+/-,34,18>)
    n511 = Multiply(x="Kp_p", y=w968) -> (x*y=w964:fxp<+/-,64,23>)
    n512 = Multiply(x="Kd_p", y=w966) -> (x*y=w965:fxp<+/-,64,27>)
    n513 = Absolute Value(x=w968) -> (abs(x)=w977:fxp<+,32,10>)
    n514 = Add(x=w964, y=w965) -> (x+y=w960:fxp<+/-,64,28>)
    n515 = Multiply(x="Ki_p", y=w962) -> (x*y=w961:fxp<+/-,64,27>)
    n516 = call "Tick Count7"() -> ("Tick Count(uSec)"=w958:u32)
    n517 = Add(x=w960, y=w961) -> (x+y=w959:fxp<+/-,64,29>)
    n518 = Greater?(x=w977, y="fp_tolorance") -> (0:w974:bool)
    n519 = Subtract(x=w958, y=w957) -> (x-y=w956:u32)
    n520 = Divide(x=u32 1000, y=w956) -> (x/y=→"PID (kHz)":fxp<+/-,20,7>)
    n521 = Select(t=w959, s=w974, f=fxp<+,1,1> 0.0) -> (s? t:f=→"Fp_PID":fxp<+/-,64,29>)
  }
  n522 = while "PD position controller_p" {
    stop <- FALSE stop-if-true
    n523 = local read "Drive mode"() -> (w980:i16)
    n524 = case shown="1" w980 {
      tunnel: [fxp<+/-,62,19> 0.0 w983] -> w979
      frame 0, Default {
        # "Backward"
      }
      frame 1 {
        # "Forward"
        n525 = local read "D_p(mm)"() -> (w990:fxp<+/-,32,7>)
        n526 = local read "Dp_error_d"() -> (w982:fxp<+/-,33,8>)
        n527 = local read "Dpr_for"() -> (w989:fxp<+/-,22,7>)
        n528 = Subtract(x=w989, y=w990) -> (x-y=w988:fxp<+/-,33,8>)
        "Dp_error" <- w988
        n529 = Multiply(x=w988, y="Kv_p") -> (x*y=w985:fxp<+/-,54,15>)
        n530 = Multiply(x=w982, y="Bv_p") -> (x*y=w984:fxp<+/-,55,16>)
        n531 = Add(x=w985, y=w984) -> (x+y=w983:fxp<+/-,55,16>)
      }
    }
    "Fr_p" <- w979
  }
  n532 = while "All switch" {
    stop <- FALSE stop-if-true
    n533 = case shown="True" "Encoder reset" {
      frame False {
        n534 = local write "Encoder reset_p"(FALSE ("Encoder reset_p")) -> ()
        n535 = local write "Encoder reset_y"(FALSE ("Encoder reset_y")) -> ()
      }
      frame True {
        n536 = flat-sequence {
          frame #0 {
            n537 = local write "Encoder reset_p"(TRUE ("Encoder reset_p")) -> ()
          }
          frame #1 {
            n538 = local write "Encoder reset_y"(TRUE ("Encoder reset_y")) -> ()
            n539 = local write "Encoder reset_p"(FALSE ("Encoder reset_p")) -> ()
          }
          frame #2 {
            n540 = local write "Encoder reset_y"(FALSE ("Encoder reset_y")) -> ()
          }
        }
      }
    }
  }
  n541 = while "Derivative" {
    stop <- FALSE stop-if-true
    n542 = local read "Dpr_sin_dd"() -> (w1007:fxp<+/-,35,20>)
    n543 = local read "Stop motor_y"() -> (w1013:bool)
    n544 = local read "Dyr_sin_dd"() -> (w1015:fxp<+/-,35,20>)
    n545 = local read "Dpr_sin_d"() -> (w1009:fxp<+/-,33,15>)
    n546 = local read "Stop motor_p"() -> (w1005:bool)
    n547 = local read "Dyr_sin_d"() -> (w1018:fxp<+/-,33,15>)
    n548 = local read "Dp_error"() -> (w1010:fxp<+/-,22,7>)
    n549 = local read "Dy_error"() -> (w1019:fxp<+/-,22,7>)
    n550 = local read "Dp_dd"() -> (w1008:fxp<+/-,36,25>)
    n551 = local read "Dy_dd"() -> (w1016:fxp<+/-,36,25>)
    n552 = Subtract(x=w1018, y=w1019) -> (x-y=w1017:fxp<+/-,34,16>)
    n553 = Subtract(x=w1015, y=w1016) -> (x-y=w1014:fxp<+/-,41,26>)
    n554 = Subtract(x=w1009, y=w1010) -> (x-y=w1002:fxp<+/-,34,16>)
    n555 = Subtract(x=w1007, y=w1008) -> (x-y=w1006:fxp<+/-,41,26>)
    n556 = Select(t=fxp<+,1,1> 0.0, s=w1013, f=w1017) -> (s? t:f=→"Dy_error_d":fxp<+/-,34,16>)
    n557 = Select(t=fxp<+/-,64,49> 0.0, s=w1013, f=w1014) -> (s? t:f=→"Dy_error_dd":fxp<+/-,64,49>)
    n558 = Select(t=fxp<+,1,1> 0.0, s=w1005, f=w1002) -> (s? t:f=→"Dp_error_d":fxp<+/-,34,16>)
    n559 = Select(t=fxp<+/-,41,26> 0.0, s=w1005, f=w1006) -> (s? t:f=→"Dp_error_dd":fxp<+/-,41,26>)
  }
  n560 = while "ft_d" {
    stop <- FALSE stop-if-true
    n561 = local read "Dy_error_dd"() -> (w1037:fxp<+/-,36,16>)
    n562 = local read "Dp_error_dd"() -> (w1028:fxp<+/-,36,16>)
    n563 = local read "Dy_error_d"() -> (w1039:fxp<+/-,33,8>)
    n564 = local read "Dp_error_d"() -> (w1030:fxp<+/-,33,8>)
    n565 = local read "Kv_p"() -> (w1031:fxp<+/-,22,8>)
    n566 = local read "Bv_p"() -> (w1029:fxp<+/-,22,8>)
    n567 = local read "Kv_y"() -> (w1040:fxp<+/-,22,8>)
    n568 = local read "Bv_y"() -> (w1038:fxp<+/-,22,8>)
    n569 = local read "Force_y"() -> (w1033:fxp<+/-,32,10>)
    n570 = Multiply(x=w1039, y=w1040) -> (x*y=w1035:fxp<+/-,55,16>)
    n571 = Multiply(x=w1037, y=w1038) -> (x*y=w1036:fxp<+/-,58,24>)
    n572 = Multiply(x=w1030, y=w1031) -> (x*y=w1026:fxp<+/-,55,16>)
    n573 = Multiply(x=w1028, y=w1029) -> (x*y=w1027:fxp<+/-,58,24>)
    n574 = local read "Force_p"() -> (w1024:fxp<+/-,32,10>)
    n575 = Add(x=w1035, y=w1036) -> (x+y=w1034:fxp<+/-,63,24>)
    n576 = Add(x=w1026, y=w1027) -> (x+y=w1025:fxp<+/-,63,24>)
    n577 = Subtract(x=w1034, y=w1033) -> (x-y=→"fyt_d":fxp<+/-,63,24>)
    n578 = Subtract(x=w1025, y=w1024) -> (x-y=→"fpt_d":fxp<+/-,63,24>)
  }
  n579 = while "Encoder_y" {
    shift-right: [w1079] -> _
    shift-left: _ -> [w1071]
    shift-right: [w1078] -> _
    shift-left: _ -> [w1070]
    shift-right: [w1069] -> _
    shift-left: _ -> [w1067]
    shift-right: [w1075] -> _
    shift-left: _ -> [w1072]
    shift-right: [w1074] -> _
    shift-left: _ -> [w1073]
    shift-right: [w1068] -> _
    shift-left: _ -> [w1066]
    stop <- FALSE stop-if-true
    w1056 = fxp<+/-,16,1> 0.0244140625  # 2*50/4096
    w1061 = fxp<+/-,20,-5> 0.00048828125  # L/4096
    w1064 = fxp<+/-,20,-5> 0.002499997615814209  # L/800
    w1046 = fxp<+/-,16,1> 0.125  # 2*50/800
    n580 = xnode "FPGA I/O Node"() -> ("Mod7/DIO2"=w1080:bool, "Mod7/DIO3"=w1081:bool)  [unwired: 2 in, 2 out]
    n581 = xnode "FPGA I/O Node"() -> ("Mod7/DIO6"=w1077:bool, "Mod7/DIO7"=w1076:bool)  [unwired: 2 in, 2 out]
    n582 = local read "Encoder reset_y"() -> (w1051:bool)
    n583 = call "encoder_sub.vi"("A_pre"=w1071, "B_pre"=w1070, "Encoder Position_pre"=w1067, "A input"=w1080, "Encoder Position Reset"="Encoder reset_y", "B input"=w1081) -> ("A"=w1079:bool, "B"=w1078:bool, "Encoder Position (Counts)"=w1069:i32)  [unwired: 19 in]
    "Encoder Position_y1" <- w1069
    n584 = call "encoder_sub.vi"("A_pre"=w1072, "B_pre"=w1073, "Encoder Position_pre"=w1066, "A input"=w1077, "Encoder Position Reset"=w1051, "B input"=w1076) -> ("A"=w1075:bool, "B"=w1074:bool, "Encoder Position (Counts)"=w1068:i32)  [unwired: 19 in]
    "Encoder Position_y2" <- w1068
    n585 = local read "Belt_in_y"() -> (w1059:fxp<+/-,6,6>)
    n586 = local read "Belt_in_y"() -> (w1063:fxp<+/-,6,6>)
    n587 = local read "Belt_out_y"() -> (w1057:fxp<+/-,7,7>)
    n588 = Divide(x=w1061, y="Mag. factor_y") -> (x/y=w1060:fxp<+/-,41,13>)
    n589 = local read "Belt_out_y"() -> (w1062:fxp<+/-,7,7>)
    n590 = To Fixed-Point(number=w1068) -> (fixed-point=w1043:fxp<+/-,32,32>)  [unwired: 1 in]
    n591 = local read "Mag. factor_y"() -> (w1055:fxp<+/-,20,3>)
    n592 = To Fixed-Point(number=w1069) -> (fixed-point=w1047:fxp<+/-,32,32>)  [unwired: 1 in]
    n593 = Multiply(x=w1060, y=w1059) -> (x*y=w1058:fxp<+/-,46,18>)
    n594 = Multiply(x=w1064, y=w1063) -> (x*y=w1065:fxp<+/-,26,1>)
    n595 = Divide(x=w1058, y=w1057) -> (x/y=w1045:fxp<+/-,53,18>)
    n596 = Divide(x=w1065, y=w1062) -> (x/y=w1049:fxp<+/-,33,1>)
    n597 = Divide(x=w1056, y=w1055) -> (x/y=w1042:fxp<+/-,37,5>)
    n598 = Multiply(x=w1045, y=w1043) -> (x*y=→"D_y2":fxp<+/-,37,7>)
    n599 = Multiply(x=w1047, y=w1046) -> (x*y=→"rad_y1":fxp<+/-,33,20>)
    n600 = Multiply(x=w1049, y=w1047) -> (x*y=→"D_y1":fxp<+/-,32,7>)
    n601 = Multiply(x=w1043, y=w1042) -> (x*y=→"rad_y2":fxp<+/-,46,16>)
  }
  n602 = while "Omega_y(T method)" {
    shift-right: [w1107] -> _
    shift-left: _ -> [w1108]
    shift-right: [w1094] -> _
    shift-left: _ -> [w1110]
    shift-right: [w1112] -> _
    shift-left: _ -> [w1113]
    shift-right: [w1085] -> _
    shift-left: _ -> [w1086]
    shift-right: [w1083] -> _
    shift-left: _ -> [w1082]
    shift-right: [w1089] -> _
    shift-left: _ -> [w1088]
    stop <- FALSE stop-if-true
    w1101 = fxp<+/-,32,0> 0.3183098859153688  # L/2/pi
    w1106 = fxp<+/-,32,0> 0.3183098859153688  # L/2/pi
    n603 = local read "Encoder Position_y1"() -> (w1107:i32)
    n604 = call "Tick Count2"() -> ("Tick Count(Ticks)"=w1087:u32)
    n605 = local read "Encoder Position_y2"() -> (w1085:i32)
    n606 = call "omega_sub_Encoder_800ppr.vi"("mt0"="mt0_y1", "omega_pre"=w1110, "ticks_m_pre"=w1113, "ticks"=w1087, "count_pre"=w1108, "count"=w1107) -> ("ticks_m"=w1112:u32, "mt"=→"mt_omega_y1":u32, "omega"=w1094:fxp<+/-,36,13>)  [unwired: 3 in]
    "omega_y1 (T)" <- w1094
    n607 = call "omega_sub_Encoder_4096ppr.vi"("mt0"="mt0_y2", "omega_pre"=w1082, "ticks_m_pre"=w1088, "ticks"=w1087, "count_pre"=w1086, "count"=w1085) -> ("ticks_m"=w1089:u32, "mt"=→"mt_omega_y2":u32, "omega"=w1083:fxp<+/-,36,13>)  [unwired: 3 in]
    n608 = local read "Belt_in_y"() -> (w1100:fxp<+/-,6,6>)
    n609 = local read "Mag. factor_y"() -> (w1102:fxp<+/-,20,3>)
    n610 = local read "Belt_out_y"() -> (w1098:fxp<+/-,7,7>)
    n611 = Multiply(x=w1106, y="Belt_in_y") -> (x*y=w1104:fxp<+/-,38,6>)
    n612 = Multiply(x=w1101, y=w1100) -> (x*y=w1099:fxp<+/-,38,6>)
    n613 = Divide(x=w1099, y=w1098) -> (x/y=w1092:fxp<+/-,45,6>)
    n614 = Divide(x=w1104, y="Belt_out_y") -> (x/y=w1095:fxp<+/-,20,1>)
    n615 = Divide(x=w1083, y=w1102) -> (x/y=w1091:fxp<+/-,57,31>)
    "omega_y2 (T)" <- w1091
    n616 = Multiply(x=w1095, y=w1094) -> (x*y=→"Dy1_d (T)":fxp<+/-,36,13>)
    n617 = Multiply(x=w1092, y=w1091) -> (x*y=→"Dy2_d (T)":fxp<+/-,36,13>)
  }
  n618 = xnode "FPGA I/O Node"("error in"=w17, "Mod6/Stop"=TRUE) -> ()  [unwired: 1 in, 2 out]
  n619 = while {
    stop <- FALSE stop-if-true
    n620 = local read "omega_y1 (Mavg)"() -> (w1122:fxp<+/-,36,14>)
    n621 = local read "omega_p1 (Mavg)"() -> (w1126:fxp<+/-,36,14>)
    n622 = local read "Dp1_d (Mavg)"() -> (w1118:fxp<+/-,36,14>)
    n623 = local read "Dy1_d (Mavg)"() -> (w1119:fxp<+/-,36,14>)
    n624 = xnode "Butterworth Filter"("input data"=w1122, "scaled coefficients"="omega_y(Mavg) coeff.") -> ("output data"=→"omega_y (Mavg w. f.)":fxp<+/-,36,18>)  [unwired: 1 in]
    n625 = xnode "Butterworth Filter"("input data"=w1126, "scaled coefficients"="omega_P(Mavg) coeff.") -> ("output data"=→"omega_p (Mavg w. f)":fxp<+/-,36,18>)  [unwired: 1 in]
    n626 = xnode "Butterworth Filter"("input data"=w1119, "scaled coefficients"="Dy_d (Mavg) coeff.") -> ("output data"=→"Dy_d (Mavg w. f.)":fxp<+/-,36,18>)  [unwired: 1 in]
    n627 = xnode "Butterworth Filter"("input data"=w1118, "scaled coefficients"="Dp_d (Mavg) coeff.") -> ("output data"=→"Dp_d (Mavg w. f.)":fxp<+/-,36,18>)  [unwired: 1 in]
  }
